vi "ME_acquire_10.vi"() -> ()   [LabVIEW 2015]
doc: "Use this template to build a producer/consumer design pattern. Use this template when you need to execute a process, such as data analysis, when a data source, such as a triggered acquisition, produces data at an uneven rate and you need to execute the process when the data becomes available."
uses:
  Mode.ctl
  oxford_driver/Oxford Drivers/BUSGEN.LLB/OxfordAddress.ctl
  <vilib>/Analysis/baseanly.llb/Mean (DBL).vi
  <vilib>/Utility/file.llb/Write Delimited Spreadsheet (DBL).vi
  <vilib>/express/express arith-compare/Formula/XNode/ExpressFormulaBlockNode.xnode
  <vilib>/Analysis/NI_AALBase.lvlib
panel:
  out "remaining elements":T1(array[cluster])
  in  "Stop":bool
  out "SaveSweep":bool=TRUE
  out "Measurement File_dn":path
  out "Measurement File_up":path
  out "Measurement File_average":path
  out "Actual Polarization":dbl
  in  "Reset IB?":bool
  in  "First?":bool
  in  "Save Period":dbl=1.0
  out "Averaged I(B)":dbl[][](array[numeric])
  out "P(uC/mm^2)":dbl[](array[numeric])
  in  "Sweep":bool
  out "P(B)":cluster{"yi":dbl[], dbl[]}(graph)
  out "Offset array":dbl[](array[numeric])
  in  "stop 2":bool
  in  "dB":dbl=0.005
  in  "Dwell Time (ms)":u32=1
  out "appended array":dbl[][](array[numeric])
  in  "Magnet ON?":bool
  out "Actual B Field (T)":dbl
  out "Actual Temperature (K)":dbl
  out "Actual Current (pA)":dbl
  in  "Tab Control":T2(tab)
  in  "Max temperature (K)":dbl=20.0
  in  "Min Temperature (K)":dbl=4.5
  out "P(T)":cluster{"yi":dbl[], dbl[]}(graph)
  out "I(T)":cluster{dbl[], dbl[]}(graph)
  in  "Set temperature (K)":dbl=4.5
  in  "Temp Ramping Rate (K/min)":dbl=10.0
  in  "Heater Range":enum16{"Off", "Low", "Medium", "High"}(ring)
  in  "Heater On/Off":bool
  out "Setpoint Temperature (K)":dbl
  in  "FileName":string
  out "Step Temp":bool
  out "j":i32
  out "i":i32
  in  "Max Countl":i32
  in  "Record ALL":bool
  in  "Sweep Rate Array":dbl[](array[numeric])=[2.0, 1.0, 0.5, 0.1, 0.05, 9.0, 10.0, 11.0, 12.0]
  out "I(B) 3":cluster{dbl[], dbl[]}[](graph)
  in  "Go to Set":bool
  in  "Set Field (T)":dbl
  in  "Field To Zero":bool
  in  "Sweep Rate (T/min)":dbl=2.0 format="%.6f"
  in  "Min Field (T)":dbl
  in  "Max Field (T)":dbl=0.15
  out "Up/Down":bool
  out "I(B) /Averaged/ 2":cluster{"B array":dbl[], dbl[]}[](graph)
  in  "Temperature Array":dbl[](array[numeric])=[4.5, 5.0, 6.0, 7.0, 8.0, 9.0, 10.0, 11.0, 12.0]
  out "New":bool=TRUE
  out "Step Rate":bool
  out "Finished":bool=TRUE
  in  "Directory":string
  out "Wait (s)":dbl
  in  "secs to wait":dbl=180.0
  in  "Max count array":i32[](array[numeric])=[2, 1, 0, 0, 0, 9, 10, 11, 12]
  in  "Measure Noise":bool
  in  "Cycles":i32
  in  "maximum value":dbl=10.0 format="%0.2f"
  in  "minimum value":dbl=-10.0 format="%0.2f"
  in  "physical channels":tag="Dev1/ai1"
  out "PSD (pA/Hz^1/2) Peaks Removed":cluster{"f0":dbl, "df":dbl, "magnitude":dbl[]}(graph)
  out "PSD (pA/Hz^1/2)":cluster{"f0":dbl, "df":dbl, "magnitude":dbl[]}(graph)
  out "Current (pA) Filtered":waveform(dbl)(graph)
  out "Current (pA)":dbl[](graph)
  in  "Samples per channel":i32=1000
  in  "Rate":dbl=1000.0 format="%0.2f"
  in  "Cut-Off Frequency":dbl=100.0 caption="Lower Cut-Off"
  in  "Filter On":bool
  out "Dc offset":dbl
  in  "Calibrate":bool
  in  "IV converter":refnum<visa-resource-name>="GPIB0::20::INSTR"
  in  "Magnetic Field":refnum<visa-resource-name>="GPIB0::21::INSTR"
  out "Time Lag":dbl=0.0500025749206543
  in  "Lake Shore":refnum<visa-resource-name>="GPIB0::11::INSTR"
  in  "Temp Refresh (s)":dbl=0.1
  in  "Sampling rate (Hz)":dbl=10.0
  in  "Gain (V/A)":dbl=1000000000.0
  in  "Sample area (mm^2)":dbl=3.9
  out "B_V":cluster{dbl[], "Best Linear Fit":dbl[]}[](graph)=[{[-0.00854253601, 0.00626134724, 0.0219834428, 0.0379117736, 0.0535871506, 0.0694316728, 0.0851615152, 0.100816481, 0.116478038, 0.132148461, 0.147876163, 0.16341701, 0.178976744, 0.194563632, 0.210251739, 0.225738944, 0.241298253, 0.256806034, 0.272344374, 0.287933477, 0.303494709, 0.318997125, 0.334591297, 0.350146681, 0.365618053, 0.380940961, 0.39666457, 0.412213675, 0.427724671, 0.443221444, 0.458760641, 0.474360042, 0.489915118, 0.505330598, 0.520967119, 0.536347531, 0.551813711, 0.567441155, 0.582995861, 0.598507522, 0.614041988, 0.629563151, 0.645106262, 0.660611914, 0.676136149, 0.691553948, 0.7071244, 0.72262999, 0.738171137, 0.753700392, 0.76919513, 0.784778028, 0.800215944, 0.8156961, 0.831325434, 0.846852183, 0.862326812, 0.877819169, 0.893312568, 0.90888536, 0.924354789], "Best Linear Fit"=[0.0, 0.005, 0.01, 0.015, 0.02, 0.025, 0.03, 0.035, 0.04, 0.045, 0.05, 0.055, 0.06, 0.065, 0.07, 0.075, 0.08, 0.085, 0.09, 0.095, 0.1, 0.105, 0.11, 0.115, 0.12, 0.125, 0.13, 0.135, 0.14, 0.145, 0.15, 0.155, 0.16, 0.165, 0.17, 0.175, 0.18, 0.185, 0.19, 0.195, 0.2, 0.205, 0.21, 0.215, 0.22, 0.225, 0.23, 0.235, 0.24, 0.245, 0.25, 0.255, 0.26, 0.265, 0.27, 0.275, 0.28, 0.285, 0.29, 0.295, 0.3]}, {[-0.00854253601, 0.00626134724, 0.0219834428, 0.0379117736, 0.0535871506, 0.0694316728, 0.0851615152, 0.100816481, 0.116478038, 0.132148461, 0.147876163, 0.16341701, 0.178976744, 0.194563632, 0.210251739, 0.225738944, 0.241298253, 0.256806034, 0.272344374, 0.287933477, 0.303494709, 0.318997125, 0.334591297, 0.350146681, 0.365618053, 0.380940961, 0.39666457, 0.412213675, 0.427724671, 0.443221444, 0.458760641, 0.474360042, 0.489915118, 0.505330598, 0.520967119, 0.536347531, 0.551813711, 0.567441155, 0.582995861, 0.598507522, 0.614041988, 0.629563151, 0.645106262, 0.660611914, 0.676136149, 0.691553948, 0.7071244, 0.72262999, 0.738171137, 0.753700392, 0.76919513, 0.784778028, 0.800215944, 0.8156961, 0.831325434, 0.846852183, 0.862326812, 0.877819169, 0.893312568, 0.90888536, 0.924354789], "Best Linear Fit"=[-0.00022554388023060128, 0.004536267537808887, 0.009593430775915074, 0.014716931562355689, 0.01975906732634002, 0.024855610270593523, 0.029915265354287977, 0.03495083565949541, 0.03998852608757118, 0.045029068349812316, 0.05008803495326229, 0.055086897848955874, 0.060091835929837946, 0.06510550835596321, 0.07015173884687344, 0.07513334727738563, 0.08013814865293042, 0.08512637555172443, 0.0901244320467579, 0.09513881694893507, 0.10014423687592358, 0.10513073807087174, 0.11014675346564809, 0.1151502923271957, 0.12012680792099008, 0.1250555686413888, 0.1301132186920259, 0.13511473785283767, 0.14010399888730068, 0.14508868495702945, 0.1500870171143548, 0.15510471446726903, 0.16010815425765457, 0.16506669165212906, 0.17009632901003072, 0.1750435864450521, 0.18001843198211442, 0.1850451496356715, 0.19004847041199868, 0.1950379453501071, 0.20003475573578386, 0.20502728708357412, 0.21002687821664084, 0.21501442030211, 0.220007939788244, 0.2249672231113706, 0.22997560874002893, 0.23496313088260184, 0.23996209027618054, 0.24495722449359253, 0.24994125598600042, 0.2549536449902534, 0.25991939913989753, 0.2648987401917687, 0.26992606578200207, 0.2749203939204135, 0.2798979571595809, 0.2848812227804405, 0.2898648235706211, 0.2948739618827834, 0.2998498524919418]}]
  out "V_I":cluster{dbl[], "Best Linear Fit":dbl[]}[](graph)=[{[0.0, 0.035, 0.069, 0.104, 0.138, 0.173, 0.208, 0.242, 0.277, 0.311, 0.346, 0.38, 0.415, 0.45, 0.484, 0.519, 0.553, 0.588, 0.623, 0.657, 0.692, 0.726, 0.761, 0.796, 0.83, 0.865, 0.899, 0.934, 0.969, 1.003, 1.038, 1.072, 1.107, 1.141, 1.176, 1.211, 1.245, 1.28, 1.314, 1.349, 1.384, 1.418, 1.453, 1.487, 1.522, 1.557, 1.591, 1.626, 1.66, 1.695, 1.73, 1.764, 1.799, 1.833, 1.868, 1.902, 1.937, 1.972, 2.006, 2.041, 2.075], "Best Linear Fit"=[-0.00854253601, 0.00626134724, 0.0219834428, 0.0379117736, 0.0535871506, 0.0694316728, 0.0851615152, 0.100816481, 0.116478038, 0.132148461, 0.147876163, 0.16341701, 0.178976744, 0.194563632, 0.210251739, 0.225738944, 0.241298253, 0.256806034, 0.272344374, 0.287933477, 0.303494709, 0.318997125, 0.334591297, 0.350146681, 0.365618053, 0.380940961, 0.39666457, 0.412213675, 0.427724671, 0.443221444, 0.458760641, 0.474360042, 0.489915118, 0.505330598, 0.520967119, 0.536347531, 0.551813711, 0.567441155, 0.582995861, 0.598507522, 0.614041988, 0.629563151, 0.645106262, 0.660611914, 0.676136149, 0.691553948, 0.7071244, 0.72262999, 0.738171137, 0.753700392, 0.76919513, 0.784778028, 0.800215944, 0.8156961, 0.831325434, 0.846852183, 0.862326812, 0.877819169, 0.893312568, 0.90888536, 0.924354789]}, {[0.0, 0.035, 0.069, 0.104, 0.138, 0.173, 0.208, 0.242, 0.277, 0.311, 0.346, 0.38, 0.415, 0.45, 0.484, 0.519, 0.553, 0.588, 0.623, 0.657, 0.692, 0.726, 0.761, 0.796, 0.83, 0.865, 0.899, 0.934, 0.969, 1.003, 1.038, 1.072, 1.107, 1.141, 1.176, 1.211, 1.245, 1.28, 1.314, 1.349, 1.384, 1.418, 1.453, 1.487, 1.522, 1.557, 1.591, 1.626, 1.66, 1.695, 1.73, 1.764, 1.799, 1.833, 1.868, 1.902, 1.937, 1.972, 2.006, 2.041, 2.075], "Best Linear Fit"=[-0.007846580254753975, 0.007882153481927697, 0.02316149482613275, 0.03889022856281441, 0.054169569907019474, 0.06989830364370113, 0.08562703738038281, 0.10090637872458785, 0.11663511246126955, 0.1319144538054746, 0.14764318754215625, 0.1629225288863613, 0.17865126262304296, 0.19437999635972467, 0.2096593377039297, 0.22538807144061138, 0.24066741278481643, 0.25639614652149806, 0.27212488025817977, 0.2874042216023848, 0.3031329553390665, 0.31841229668327153, 0.3341410304199532, 0.3498697641566349, 0.3651491055008399, 0.3808778392375216, 0.39615718058172666, 0.4118859143184083, 0.42761464805509, 0.442893989399295, 0.45862272313597674, 0.4739020644801818, 0.48963079821686345, 0.5049101395610684, 0.5206388732977502, 0.5363676070344319, 0.5516469483786369, 0.5673756821153185, 0.5826550234595236, 0.5983837571962053, 0.6141124909328869, 0.629391832277092, 0.6451205660137737, 0.6603999073579787, 0.6761286410946604, 0.691857374831342, 0.7071367161755471, 0.7228654499122288, 0.7381447912564338, 0.7538735249931156, 0.7696022587297972, 0.7848816000740022, 0.8006103338106839, 0.815889675154889, 0.8316184088915707, 0.8468977502357756, 0.8626264839724573, 0.878355217709139, 0.893634559053344, 0.9093632927900257, 0.9246426341342309]}]
  out "B0 (T)":dbl=0.0025222449819540214
  out "B/V (T/V)":dbl=0.321659617116981
  out "I0 (A)":dbl=-0.007846580254753975
  out "V/I (Ohm)":dbl=0.44939239247661916
  in  "Offset?":bool
  in  "Temp/Magnetic Field":bool
  out "index":i8
  out "Read?":bool
  out "Magnetic Field (T)":dbl[](array[numeric])
  out "Reset":bool
  out "Measured Current (pA)":dbl[](array[numeric])
  out "Elapsed Time (s)":dbl[](array[numeric])
  out "Start time":timestamp
  in  "Enum":T3=enum."Process"
  out "B array":dbl[](array[numeric])
  in  "dB (T)":dbl=0.0025
  in  "Counter":i8
  out "L magnet (H)":dbl
  out "R magnet (mOhm)":dbl
  out "Actual Current (R0)":dbl
  out "Actual Field (T)":dbl
  out "Temperature array":dbl[](array[numeric])
  in  "New Measurement File":bool
  out "Measurement File":path
  out "refnum out":refnum<file>
  in  "Measuring":bool
  in  "Measure /Pause":bool
  in  "stop":bool
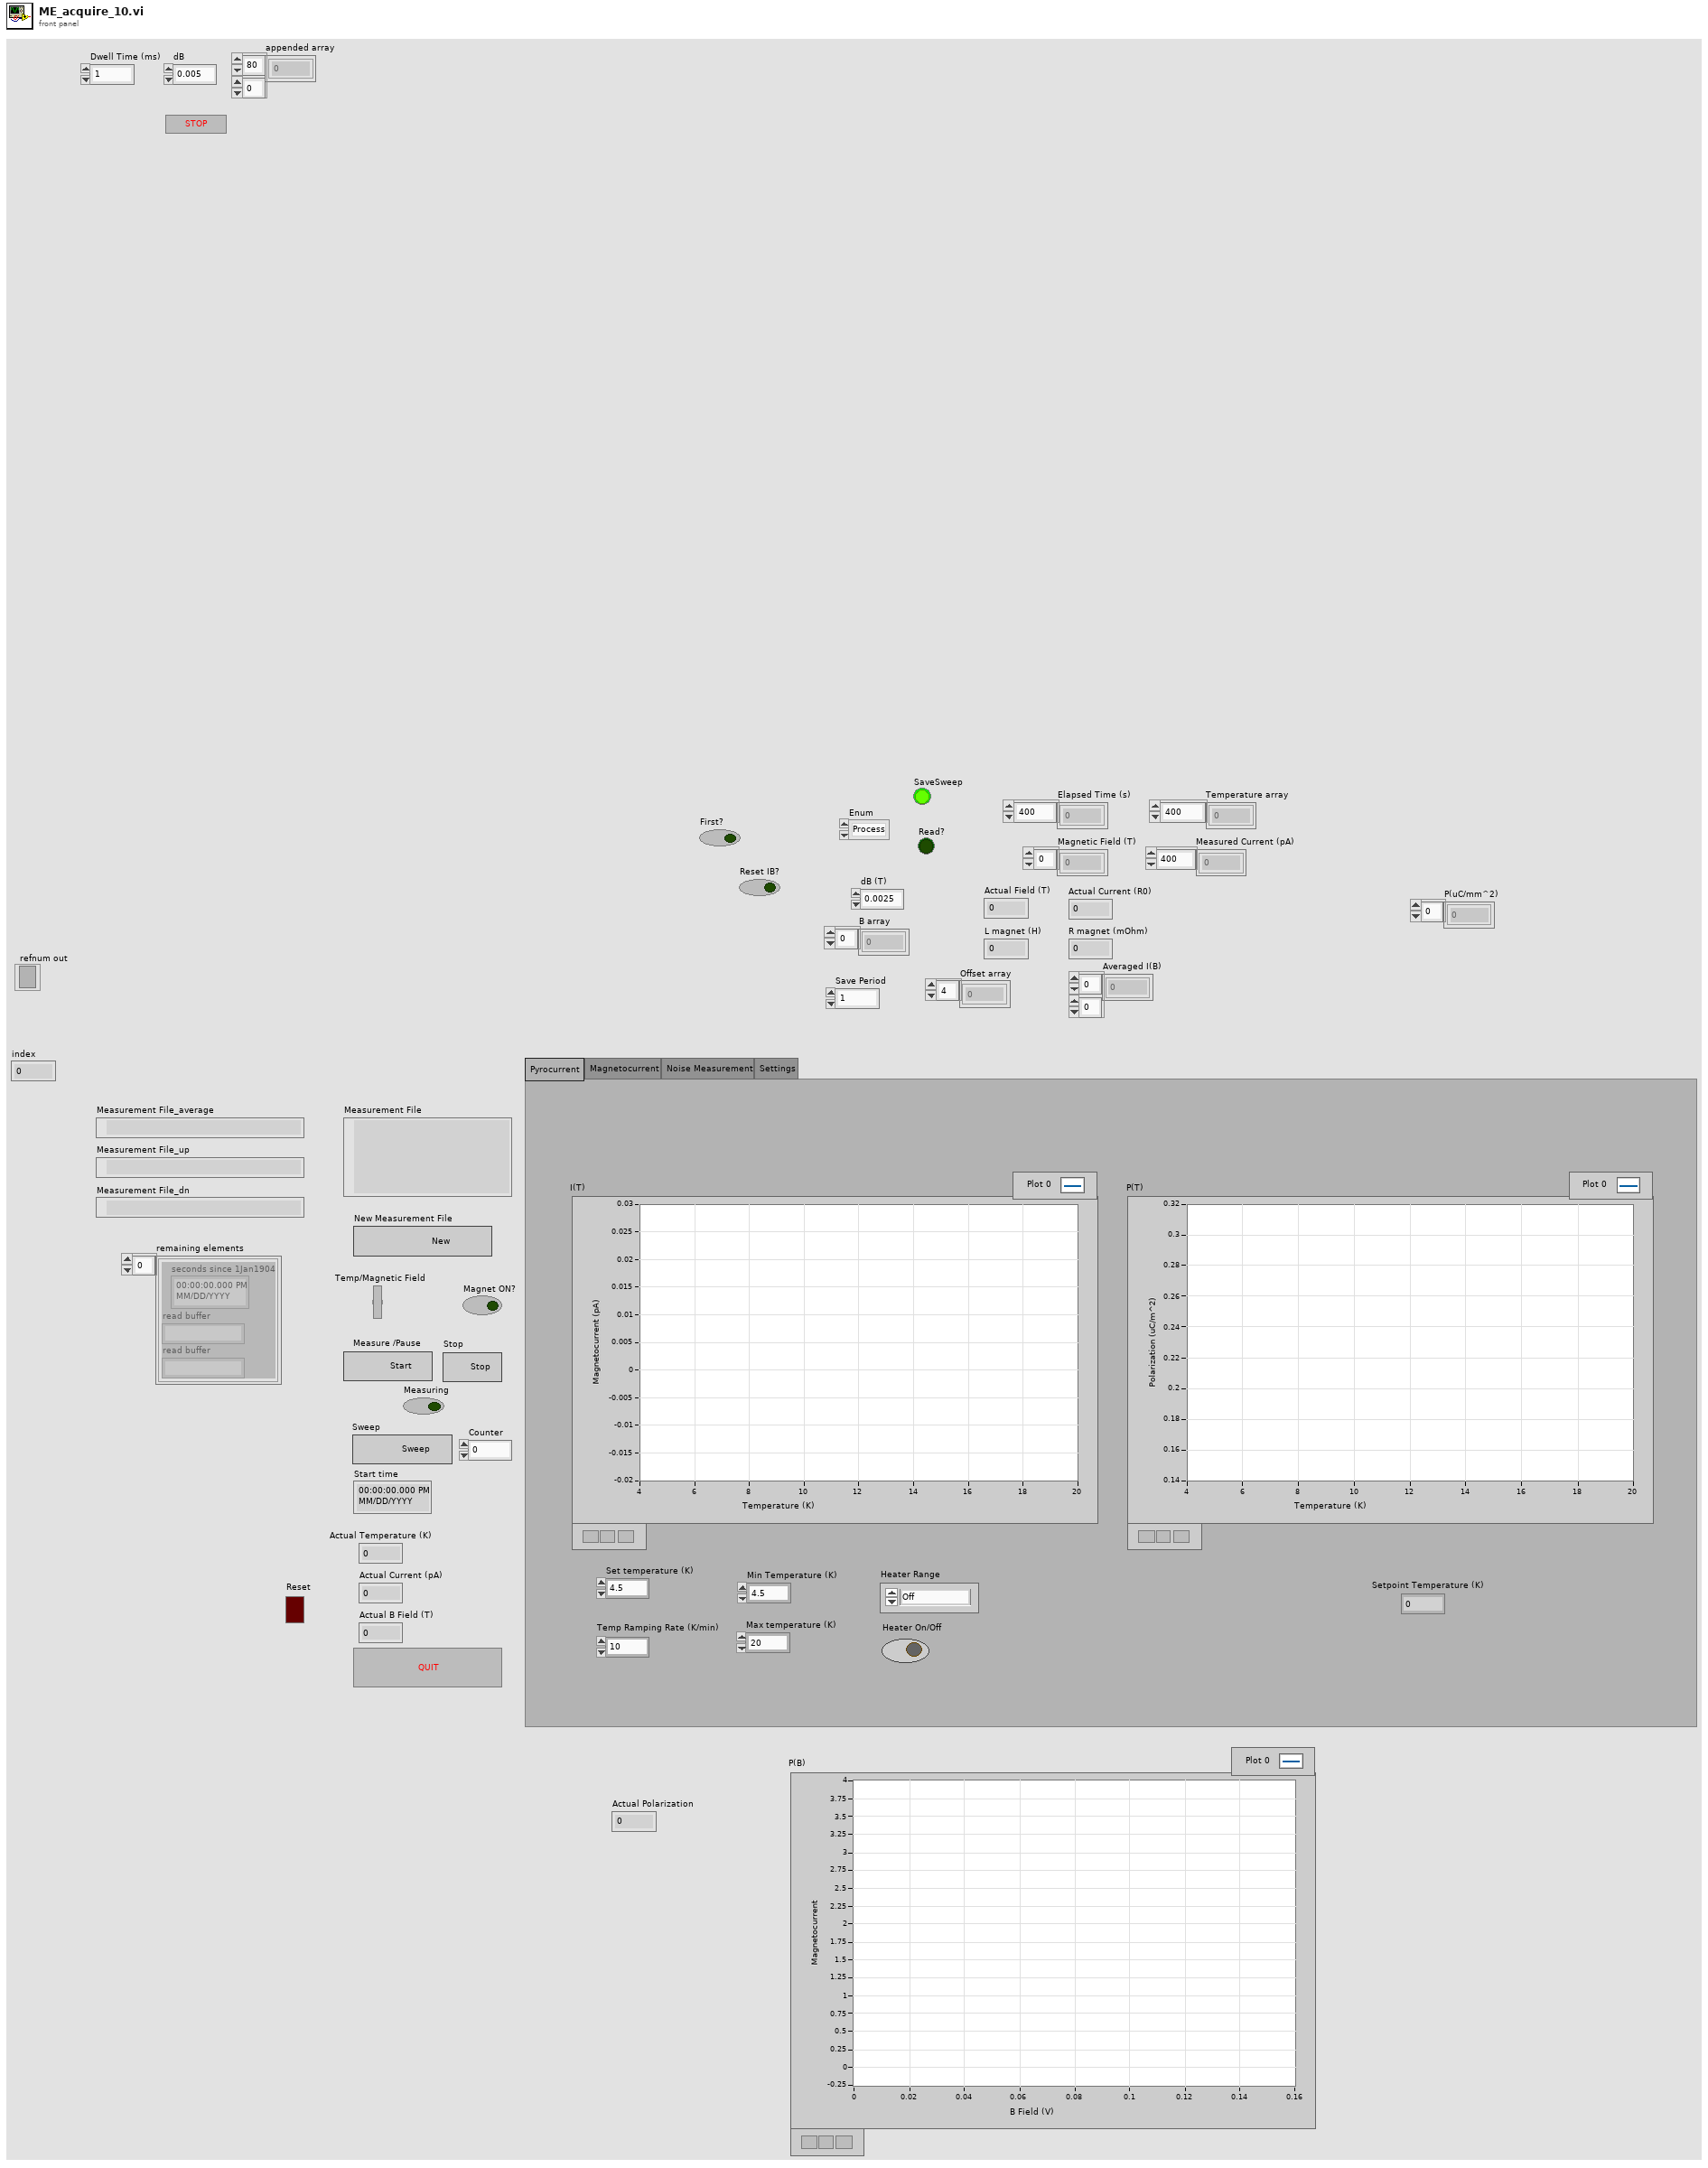
[diagram p1: front panel]
types:
  T1 = cluster{"seconds since 1Jan1904":timestamp, "read buffer":string, "read buffer":string}[]
  T2 = enum32{"Pyrocurrent", "Magnetocurrent", "Noise Measurement", "Settings"}
  T3 = typedef "Mode.ctl" = enum16{"Offset", "Process", "Sweep", "Plot", "Save", "New", "Return", ""}
  T4 = enum16{"open", "replace", "create", "open or create", "replace or create", "replace or create with confirmation"}
  T5 = typedef "OxfordAddress.ctl" = cluster{"Com Port":i32, "ISOBUS Address":i32, "GPIB Address":i16, "Communication":enum16{"RS232", "ISOBUS", "GPIB", "Gateway"}}
  T6 = cluster{"seconds since 1Jan1904":timestamp, "read buffer":string, "read buffer":string}
  T7 = cluster{"B array":dbl[], "Averaged I(B) out":dbl[]}
  T8 = cluster{"B array":dbl[], "Averaged I(B) out":dbl[]}[]
  T9 = cluster{"I array out (A)":dbl[], "V array out (V)":dbl[]}
  T10 = cluster{"I array out (A)":dbl[], "Best Linear Fit":dbl[]}
  T11 = cluster{"V array out (V)":dbl[], "B array Out":dbl[]}
  T12 = cluster{"V array out (V)":dbl[], "Best Linear Fit 2":dbl[]}
  T13 = cluster{"I array out (A)":dbl[], "Best Linear Fit":dbl[]}[]
  T14 = cluster{"V array out (V)":dbl[], "Best Linear Fit 2":dbl[]}[]
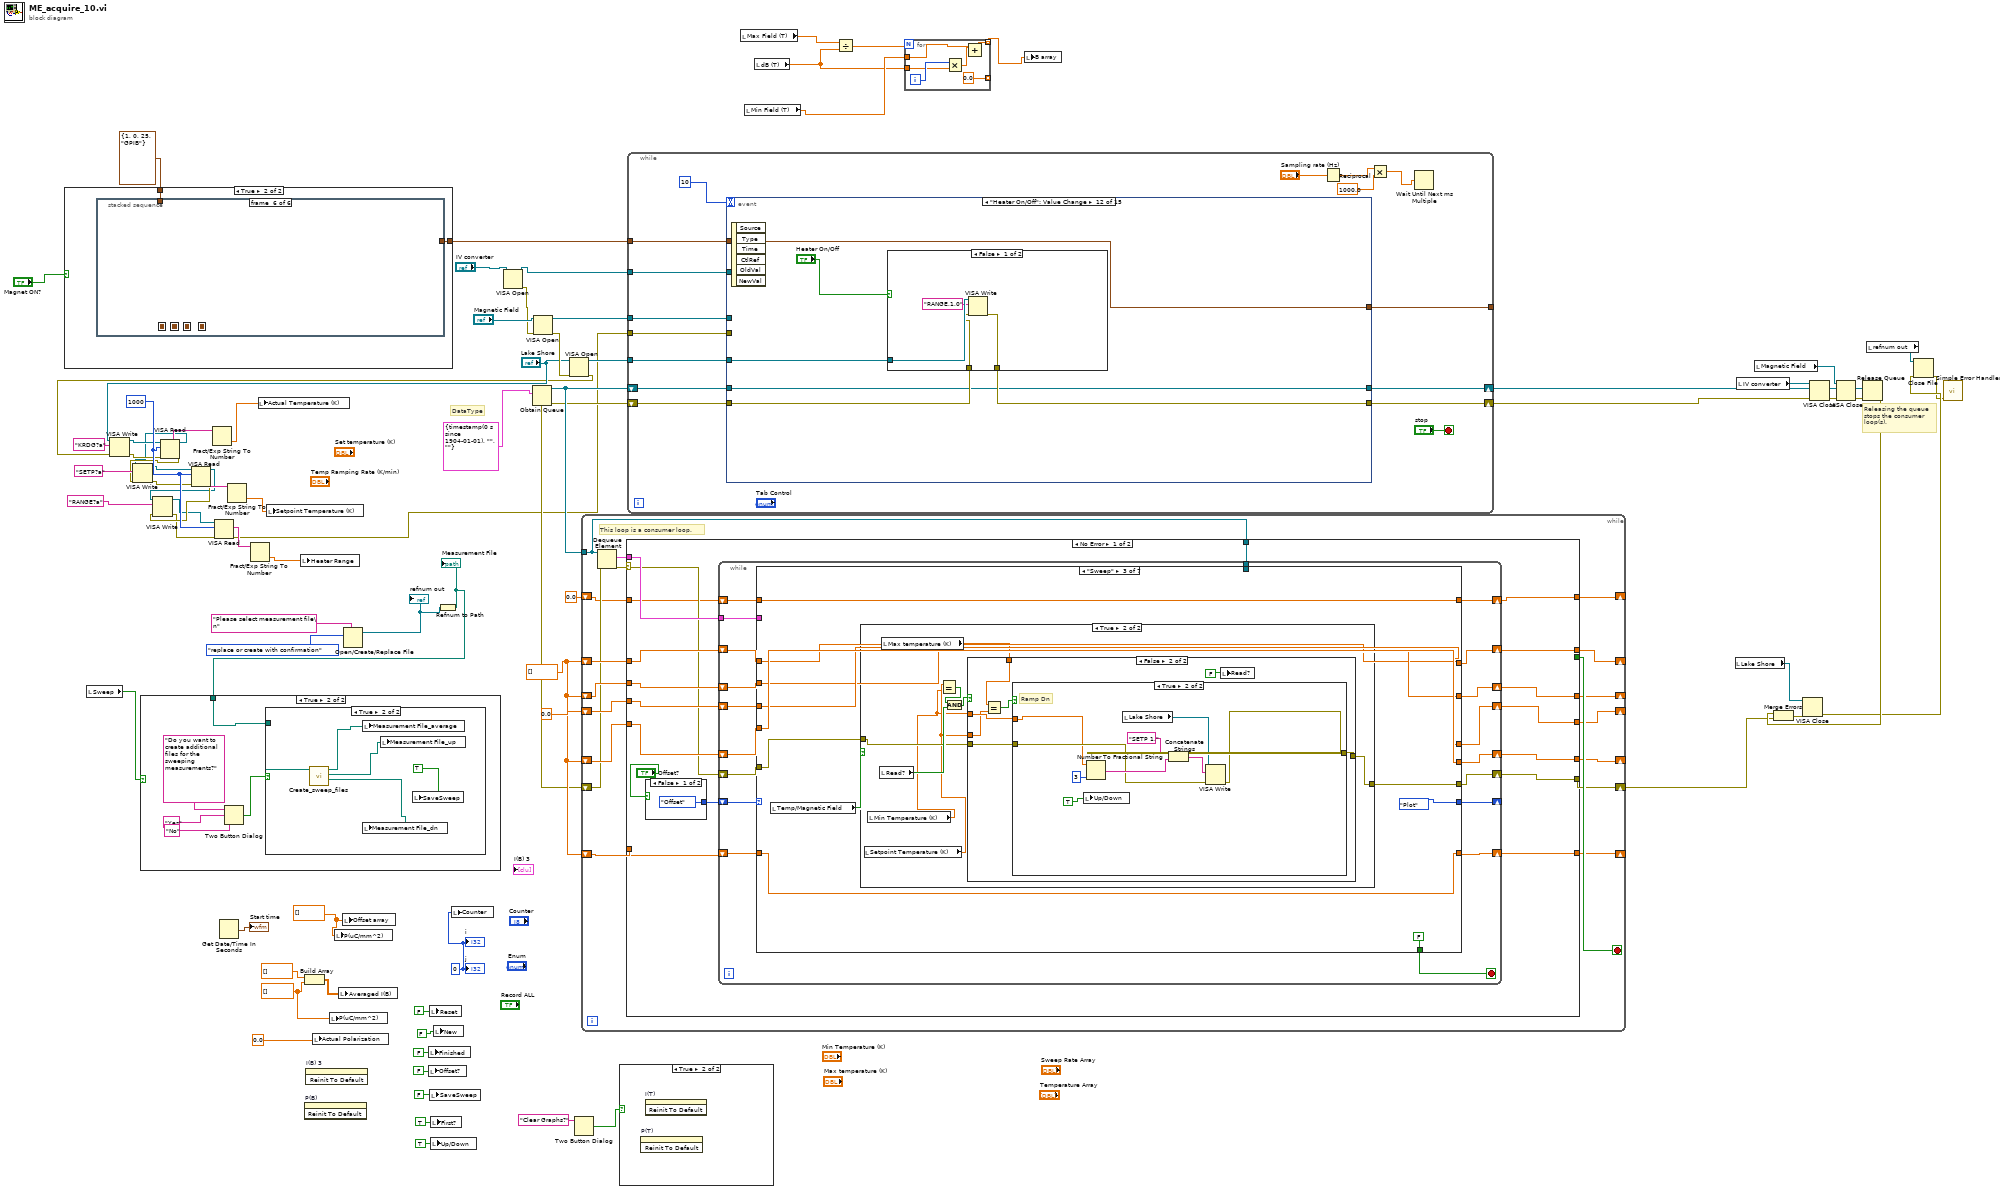
[diagram p0: block diagram]
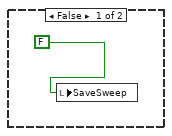
[diagram p4: hidden frame]
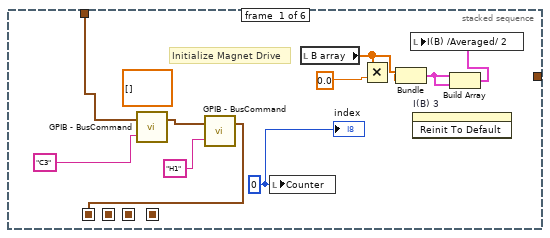
[diagram p6: hidden frame]
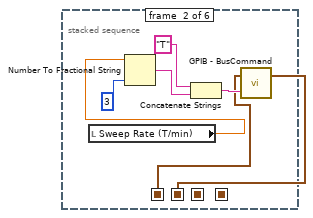
[diagram p7: hidden frame]
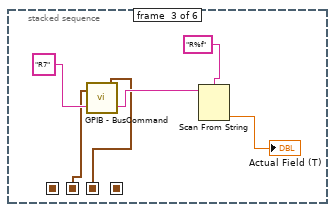
[diagram p8: hidden frame]
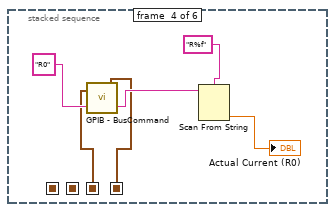
[diagram p9: hidden frame]
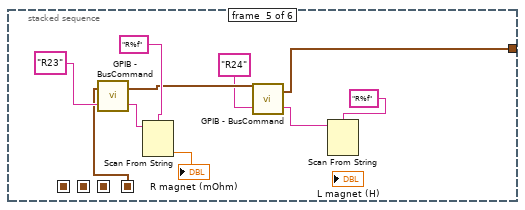
[diagram p10: hidden frame]
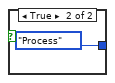
[diagram p11: hidden frame]
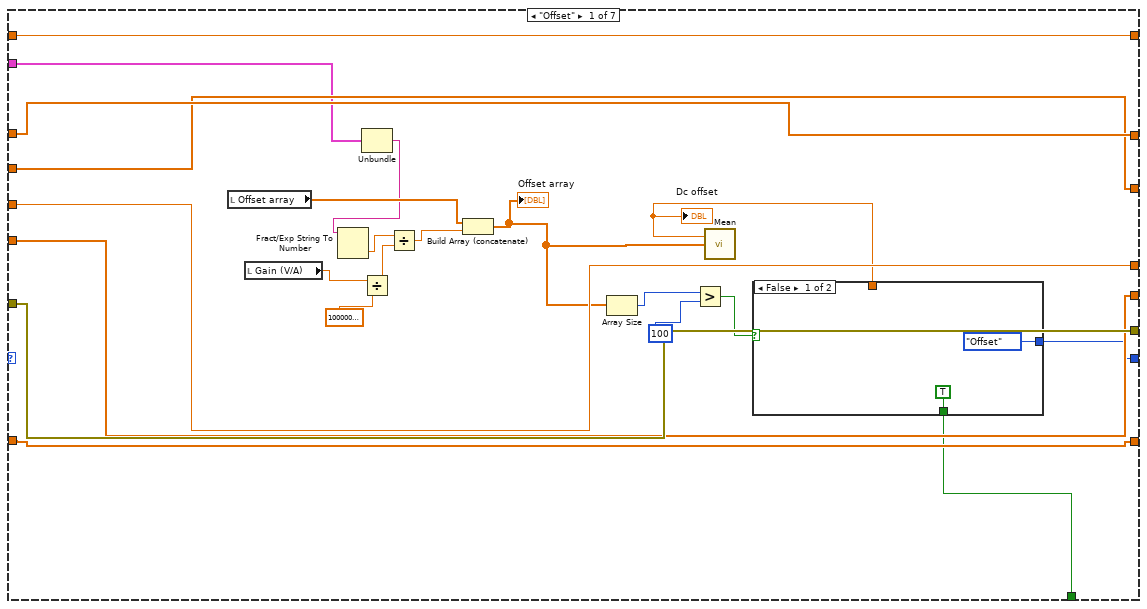
[diagram p12: hidden frame]
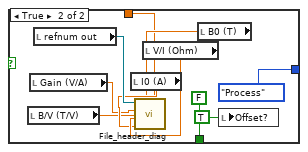
[diagram p13: hidden frame]
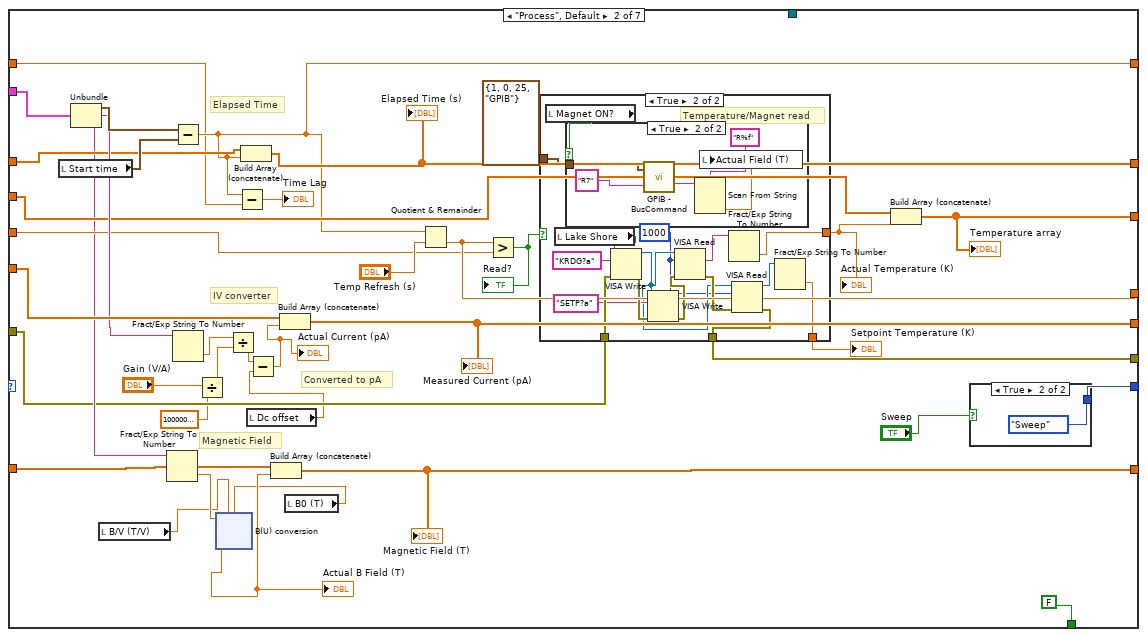
[diagram p14: hidden frame]
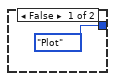
[diagram p15: hidden frame]
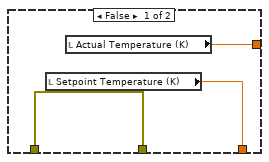
[diagram p16: hidden frame]
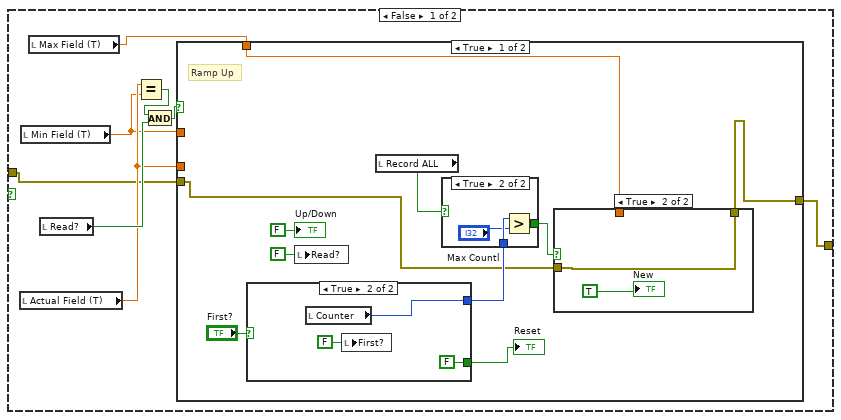
[diagram p18: hidden frame]
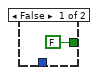
[diagram p19: hidden frame]
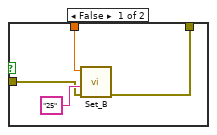
[diagram p20: hidden frame]
diagram:
  w16 = u32 1000 ("byte count")
  w27 = 0 ("j")
  w24 = dbl[] []
  w45 = dbl[] []
  w51 = dbl[] []
  # "DataType"
  # "Releasing the queue stops the consumer loop(s)."
  n1 = case shown="True" "Magnet ON?" {
    tunnel: T5 {"Com Port"=1, "ISOBUS Address"=0, "GPIB Address"=25, "Communication"=enum."GPIB"} ("Address") -> [w79 w81]
    tunnel: [w79 w80] -> w58
    frame False {
    }
    frame True {
      n2 = stacked-sequence {
        seq-local: [w89 _ _ _ _ _] -> [_ w94 _ _ _ _]
        seq-local: [_ w93 _ _ _ _] -> [_ _ w101 _ _ _]
        seq-local: [_ _ w100 _ _ _] -> [_ _ _ w107 _ _]
        seq-local: [_ _ _ w106 _ _] -> [_ _ _ _ w117 _]
        tunnel: w81 -> [w91 _ _ _ _ _]
        tunnel: [_ _ _ _ w115 _] -> w80
        frame #0 {
          (unwired) dbl[][] []
          w87 = i8 0 ("Counter")
          # "Initialize Magnet Drive"
          n3 = call "GPIB - BusCommand.vi"("Command"="C3", "Address"=w91) -> ("Address(thru)"=w90:T5)  [unwired: 1 out]
          n4 = call "GPIB - BusCommand.vi"("Command"="H1", "Address"=w90) -> ("Address(thru)"=w89:T5)  [unwired: 1 out]
          n5 = local write "Counter"(w87) -> ()
          n6 = local read "B array"() -> (w85:dbl[])
          n7 = Multiply(x=w85, y=0.0) -> (x*y=w84:dbl[])
          n8 = Bundle("B array"=w85, w84) -> (w83:cluster{"B array":dbl[], dbl[]})  [unwired: 1 in]
          n9 = invoke on="I(B) 3" class="XYGraph (strict)" method="Reinit To Default"() -> ()  [unwired: 3 in, 3 out]
          n10 = Build Array(w83, w83) -> (w82:cluster{"B array":dbl[], dbl[]}[])
          n11 = local write "I(B) /Averaged/ 2"(w82) -> ()
          "index" <- w87
        }
        frame #1 {
          n12 = local read "Sweep Rate (T/min)"() -> (w95:dbl)
          n13 = Number To Fractional String(number=w95, precision (6)=i16 3) -> (F-format string=w97:string)  [unwired: 2 in]
          n14 = Concatenate Strings("T" ("format string"), w97) -> (w96:string)
          n15 = call "GPIB - BusCommand.vi"("Command"=w96, "Address"=w94) -> ("Address(thru)"=w93:T5)  [unwired: 1 out]
        }
        frame #2 {
          n16 = call "GPIB - BusCommand.vi"("Command"="R7" ("format string"), "Address"=w101) -> ("Reply"=w105:string, "Address(thru)"=w100:T5)
          n17 = Scan From String(format string="R%f" ("remaining string"), input string=w105) -> (output 1=→"Actual Field (T)":dbl)  [unwired: 3 in, 3 out]
        }
        frame #3 {
          n18 = call "GPIB - BusCommand.vi"("Command"="R0" ("format string"), "Address"=w107) -> ("Reply"=w111:string, "Address(thru)"=w106:T5)
          n19 = Scan From String(format string="R%f" ("remaining string"), input string=w111) -> (output 1=→"Actual Current (R0)":dbl)  [unwired: 3 in, 3 out]
        }
        frame #4 {
          n20 = call "GPIB - BusCommand.vi"("Command"="R23" ("format string"), "Address"=w117) -> ("Reply"=w121:string, "Address(thru)"=w116:T5)
          n21 = Scan From String(format string="R%f" ("remaining string"), input string=w121) -> (output 1=→"R magnet (mOhm)":dbl)  [unwired: 3 in, 3 out]
          n22 = call "GPIB - BusCommand.vi"("Command"="R24" ("format string"), "Address"=w116) -> ("Reply"=w113:string, "Address(thru)"=w115:T5)
          n23 = Scan From String(format string="R%f" ("remaining string"), input string=w113) -> ()  [unwired: 4 in, 3 out]
        }
        frame #5 {
        }
      }
    }
  }
  n24 = local read "Sweep"() -> (w32:bool)
  n25 = Get Date/Time In Seconds() -> (seconds since 1Jan1904=→"Start time":timestamp)
  n26 = Build Array(dbl[] [], w24) -> (w43:dbl[][])
  n27 = invoke on="P(B)" class="XYGraph (strict)" method="Reinit To Default"() -> ()  [unwired: 3 in, 3 out]
  n28 = invoke on="I(B) 3" class="XYGraph (strict)" method="Reinit To Default"() -> ()  [unwired: 3 in, 3 out]
  n29 = local write "Actual Polarization"(0.0 ("Actual Polarization")) -> ()
  n30 = local write "P(uC/mm^2)"(w24) -> ()
  n31 = local write "P(uC/mm^2)"(w45) -> ()
  n32 = local write "Averaged I(B)"(w43) -> ()
  n33 = local write "Offset array"(w45) -> ()
  n34 = Open/Create/Replace File(prompt="Please select measurement file\n", operation (0:open)=T4."replace or create with confirmation") -> (refnum out=w55:refnum<file>)  [unwired: 4 in, 2 out]
  "refnum out" <- w55
  n35 = local write "Finished"(FALSE ("Finished")) -> ()
  n36 = local write "Offset?"(FALSE ("Offset?")) -> ()
  n37 = local write "Reset"(FALSE ("Reset")) -> ()
  n38 = local write "SaveSweep"(FALSE ("SaveSweep")) -> ()
  n39 = local write "First?"(TRUE ("First?")) -> ()
  n40 = local write "Up/Down"(TRUE ("Up/Down")) -> ()
  n41 = local write "New"(FALSE ("New")) -> ()
  n42 = Refnum to Path(1:w55) -> (0:w31:path)
  "Measurement File" <- w31
  n43 = case shown="True" w32 {
    tunnel: w31 -> [_ w122]
    frame False {
    }
    frame True {
      n44 = Two Button Dialog(message="Do you want to create additional files for the sweeping measurements?" ("string"), 1:"No" ("F button name (\"Cancel\")"), 2:"Yes" ("T button name (\"OK\")")) -> (T button?=w124:bool)
      n45 = case shown="True" w124 {
        tunnel: w122 -> [_ w132]
        frame False {
          n46 = local write "SaveSweep"(FALSE ("SaveSweep")) -> ()
        }
        frame True {
          n47 = call "Create_sweep_files.vi"("Measurement File"=w132) -> ("Path 3"=w129:path, "Path 2"=w130:path, "Path"=w131:path)  [unwired: 8 in]
          n48 = local write "Measurement File_dn"(w129) -> ()
          n49 = local write "Measurement File_average"(w131) -> ()
          n50 = local write "Measurement File_up"(w130) -> ()
          n51 = local write "SaveSweep"(TRUE) -> ()
        }
      }
    }
  }
  n52 = local write "Counter"(w27) -> ()
  n53 = VISA Open(VISA resource name="IV converter") -> (VISA resource name=w73:refnum<visa-resource-name>, error out=w75:errorcluster)  [unwired: 4 in]
  n54 = Obtain Queue(element data type=T6 {"seconds since 1Jan1904"=timestamp(0 s since 1904-01-01), "read buffer"="", "read buffer"=""} ("output cluster")) -> (queue out=w78:refnum<queue>, error out=w49:errorcluster)  [unwired: 4 in, 1 out]
  n55 = VISA Open(error in (no error)=w75, VISA resource name="Magnetic Field") -> (VISA resource name=w72:refnum<visa-resource-name>, error out=w52:errorcluster)  [unwired: 3 in]
  n56 = VISA Open(error in (no error)=w52, VISA resource name="Lake Shore") -> (VISA resource name=w47:refnum<visa-resource-name>, error out=w13:errorcluster)  [unwired: 3 in]
  n57 = VISA Write(VISA resource name="Lake Shore", write buffer="KRDG?a", error in (no error)=w13) -> (VISA resource name out=w10:refnum<visa-resource-name>, error out=w9:errorcluster)  [unwired: 1 out]
  n58 = VISA Read(VISA resource name=w10, byte count=w16, error in (no error)=w9) -> (VISA resource name out=w7:refnum<visa-resource-name>, read buffer=w21:string, error out=w8:errorcluster)  [unwired: 1 out]
  n59 = VISA Write(VISA resource name=w7, write buffer="SETP?a", error in (no error)=w8) -> (VISA resource name out=w6:refnum<visa-resource-name>, error out=w5:errorcluster)  [unwired: 1 out]
  n60 = VISA Read(VISA resource name=w6, byte count=w16, error in (no error)=w5) -> (VISA resource name out=w3:refnum<visa-resource-name>, read buffer=w20:string, error out=w4:errorcluster)  [unwired: 1 out]
  n61 = VISA Write(VISA resource name=w3, write buffer="RANGE?a", error in (no error)=w4) -> (VISA resource name out=w1:refnum<visa-resource-name>, error out=w2:errorcluster)  [unwired: 1 out]
  n62 = Fract/Exp String To Number(string=w21) -> (number=w19:dbl)  [unwired: 3 in, 1 out]
  n63 = VISA Read(VISA resource name=w1, byte count=w16, error in (no error)=w2) -> (read buffer=w15:string, error out=w12:errorcluster)  [unwired: 2 out]
  n64 = Fract/Exp String To Number(string=w20) -> (number=w18:dbl)  [unwired: 3 in, 1 out]
  n65 = Fract/Exp String To Number(string=w15) -> (number=w11:dbl)  [unwired: 3 in, 1 out]
  n66 = local write "Actual Temperature (K)"(w19) -> ()
  n67 = local write "Setpoint Temperature (K)"(w18) -> ()
  n68 = local write "Heater Range"(w11) -> ()
  n69 = Two Button Dialog(message="Clear Graphs?") -> (T button?=w26:bool)  [unwired: 2 in]
  n70 = while {
    tunnel: w78 -> [w133]
    shift-right: [w146] -> _
    shift-left: w51 -> [w145]
    shift-right: [w144] -> _
    shift-left: w51 -> [w143]
    shift-right: [w142] -> _
    shift-left: w51 -> [w141]
    shift-right: [w140] -> _
    shift-left: 0.0 -> [w139]
    shift-right: [w138] -> _
    shift-left: w51 -> [w137]
    shift-right: [w147] -> w63
    shift-left: w49 -> [w136]
    shift-right: [w135] -> _
    shift-left: 0.0 -> [w134]
    stop <- w148 stop-if-true
    # "This loop is a consumer loop."
    n71 = Dequeue Element(queue=w133, error in (no error)=w136) -> (element=w149:T6, error out=w150:errorcluster)  [unwired: 1 in, 2 out]
    n72 = case shown="No Error" w150 {
      selector: w150 -> [w156 w714]
      tunnel: w149 -> [w167 _]
      tunnel: [_ TRUE] -> w148
      tunnel: [w155 w714] -> w147
      tunnel: [w166 w713] -> w146
      tunnel: w145 -> [w165 w713]
      tunnel: [w164 w710] -> w144
      tunnel: w143 -> [w163 w710]
      tunnel: [w162 w709] -> w142
      tunnel: w141 -> [w161 w709]
      tunnel: [w160 w711] -> w140
      tunnel: w139 -> [w159 w711]
      tunnel: [w158 w712] -> w138
      tunnel: w137 -> [w157 w712]
      tunnel: [w154 w708] -> w135
      tunnel: w134 -> [w153 w708]
      tunnel: w133 -> [w151 _]
      frame No Error {
        n73 = case shown="False" "Offset?" {
          tunnel: [Mode."Offset" ("Enum") Mode."Process" ("Enum")] -> w168
          frame False {
          }
          frame True {
          }
        }
        n74 = while {
          shift-right: [w177] -> _
          shift-left: w168 -> [w189]
          tunnel: w167 -> [w188]
          shift-right: [w187] -> w166
          shift-left: w165 -> [w186]
          shift-right: [w179] -> w158
          shift-left: w157 -> [w178]
          shift-right: [w181] -> w160
          shift-left: w159 -> [w180]
          shift-right: [w185] -> w164
          shift-left: w163 -> [w184]
          shift-right: [w175] -> w155
          shift-left: w156 -> [w176]
          shift-right: [w183] -> w162
          shift-left: w161 -> [w182]
          shift-right: [w173] -> w154
          shift-left: w153 -> [w172]
          tunnel: w151 -> [w171]
          stop <- w174 stop-if-true
          n75 = case shown="\"Sweep\"" w189 {
            selector: w189 -> [_ _ _ _ _ _ w701]
            tunnel: w188 -> [w205 w260 _ _ _ _ _]
            tunnel: [w211 w257 w304 w409 w482 w550 w706] -> w187
            tunnel: w186 -> [w211 w248 w304 w409 w478 w550 w706]
            tunnel: [w206 w256 w307 w411 w484 w548 w703] -> w185
            tunnel: w184 -> [w206 w255 w307 w411 w479 w548 w703]
            tunnel: [w207 w252 w309 w406 w485 w546 w700] -> w183
            tunnel: w182 -> [w207 w251 w309 w406 w480 w546 w700]
            tunnel: [w209 w247 w306 w407 w488 0.0 w704] -> w181
            tunnel: w180 -> [w209 w246 w306 w407 w488 _ w704]
            tunnel: [w210 w243 w305 w408 w483 w549 w705] -> w179
            tunnel: w178 -> [w210 w244 w305 w408 w481 w549 w705]
            tunnel: [w194 w241 Mode."Plot" ("Enum") Mode."Save" ("Enum") w489 Mode."Return" ("Enum") w701] -> w177
            tunnel: w176 -> [w208 w239 w311 w414 w487 w542 w702]
            tunnel: [w208 w238 w310 w414 w487 w541 w702] -> w175
            tunnel: [w190 FALSE FALSE FALSE w476 TRUE TRUE] -> w174
            tunnel: [w193 w235 w303 w410 w486 0.0 w707] -> w173
            tunnel: w172 -> [w193 w234 w303 w410 w486 _ w707]
            tunnel: w171 -> [_ _ _ _ _ w540 _]
            frame "Offset" {
              n76 = local read "Offset array"() -> (w199:dbl[])
              n77 = local read "Gain (V/A)"() -> (w203:dbl)
              n78 = Unbundle(w205) -> ("read buffer"=w192:string)  [unwired: 2 out]
              n79 = Fract/Exp String To Number(string=w192) -> (number=w204:dbl)  [unwired: 3 in, 1 out]
              n80 = Divide(x=w203, y=1000000000000.0) -> (x/y=w201:dbl)
              n81 = Divide(x=w204, y=w201) -> (x/y=w200:dbl)
              n82 = Build Array (concatenate)(w199, w200) -> (w195:dbl[])
              "Offset array" <- w195
              n83 = Array Size(array=w195) -> (size(s)=w198:i32)
              n84 = Greater?(x=w198, y=100) -> (0:w196:bool)
              n85 = call-poly <vilib>:"Mean.vi"("X"=w195) -> ("mean"=w191:dbl)  [unwired: 1 out]
              "Dc offset" <- w191
              n86 = case shown="False" w196 {
                tunnel: [Mode."Offset" ("Enum") Mode."Process" ("Enum")] -> w194
                tunnel: w191 -> [_ w215]
                tunnel: [TRUE FALSE] -> w190
                frame False {
                }
                frame True {
                  n87 = local read "B/V (T/V)"() -> (w216:dbl)
                  n88 = local read "Gain (V/A)"() -> (w217:dbl)
                  n89 = local read "refnum out"() -> (w221:refnum<file>)
                  n90 = local read "I0 (A)"() -> (w219:dbl)
                  n91 = local read "V/I (Ohm)"() -> (w220:dbl)
                  n92 = local read "B0 (T)"() -> (w218:dbl)
                  n93 = call "File_header_diag.vi"("OFFSET"=w215, "B0"=w218, "B/V"=w216, "I0"=w219, "V/I"=w220, "Gain"=w217, "Byte Stream File in"=w221) -> ()  [unwired: 5 in]
                  n94 = local write "Offset?"(TRUE ("Offset?")) -> ()
                }
              }
            }
            frame "Process", Default {
              # "Converted to pA"
              # "Magnetic Field"
              # "IV converter"
              # "Elapsed Time"
              n95 = local read "Start time"() -> (w258:timestamp)
              n96 = Unbundle(w260) -> ("seconds since 1Jan1904"=w259:timestamp, "read buffer"=w253:string, "read buffer"=w240:string)
              n97 = local read "B/V (T/V)"() -> (w230:dbl)
              n98 = Fract/Exp String To Number(string=w240) -> (number=w250:dbl)  [unwired: 3 in, 1 out]
              n99 = Subtract(x=w259, y=w258) -> (x-y=w235:dbl)
              n100 = Fract/Exp String To Number(string=w253) -> (number=w254:dbl)  [unwired: 3 in, 1 out]
              n101 = Divide(x="Gain (V/A)", y=1000000000000.0) -> (x/y=w233:dbl)
              n102 = Divide(x=w254, y=w233) -> (x/y=w228:dbl)
              n103 = Subtract(x=w235, y=w234) -> (x-y=→"Time Lag":dbl)
              n104 = Build Array (concatenate)(w248, w235) -> (w257:dbl[])
              "Elapsed Time (s)" <- w257
              n105 = local read "Dc offset"() -> (w226:dbl)
              n106 = Subtract(x=w228, y=w226) -> (x-y=w227:dbl)
              "Actual Current (pA)" <- w227
              n107 = Build Array (concatenate)(w255, w227) -> (w256:dbl[])
              "Measured Current (pA)" <- w256
              n108 = local read "B0 (T)"() -> (w229:dbl)
              n109 = xnode "B(U) conversion"("V"=w250, "BpV"=w230, "B0"=w229) -> ("Result"=w249:dbl)  [unwired: 1 in, 1 out]
              "Actual B Field (T)" <- w249
              n110 = Build Array (concatenate)(w251, w249) -> (w252:dbl[])
              "Magnetic Field (T)" <- w252
              n111 = Quotient & Remainder(x=w235, y="Temp Refresh (s)") -> (floor(x/y)=w247:dbl)  [unwired: 1 out]
              n112 = Greater?(x=w247, y=w246) -> (0:w245:bool)
              "Read?" <- w245
              n113 = case shown="True" w245 {
                tunnel: [w266 w281] -> w242
                tunnel: w239 -> [w267 w280]
                tunnel: [w267 w272] -> w238
                tunnel: T5 {"Com Port"=1, "ISOBUS Address"=0, "GPIB Address"=25, "Communication"=enum."GPIB"} ("Address") -> [_ w279]
                tunnel: [w265 w268] -> w224
                frame False {
                  n114 = local read "Setpoint Temperature (K)"() -> (w265:dbl)
                  n115 = local read "Actual Temperature (K)"() -> (w266:dbl)
                }
                frame True {
                  w270 = u32 1000 ("byte count")
                  # "Temperature/Magnet read"
                  n116 = local read "Magnet ON?"() -> (w277:bool)
                  n117 = local read "Lake Shore"() -> (w278:refnum<visa-resource-name>)
                  n118 = case shown="True" w277 {
                    tunnel: w279 -> [_ w285]
                    frame False {
                    }
                    frame True {
                      n119 = call "GPIB - BusCommand.vi"("Command"="R7" ("format string"), "Address"=w285) -> ("Reply"=w286:string)  [unwired: 1 out]
                      n120 = Scan From String(format string="R%f" ("remaining string"), input string=w286) -> (output 1=w284:dbl)  [unwired: 3 in, 3 out]
                      n121 = local write "Actual Field (T)"(w284) -> ()
                    }
                  }
                  n122 = VISA Write(VISA resource name=w278, write buffer="KRDG?a", error in (no error)=w280) -> (VISA resource name out=w271:refnum<visa-resource-name>, error out=w276:errorcluster)  [unwired: 1 out]
                  n123 = VISA Write(VISA resource name=w271, write buffer="SETP?a", error in (no error)=w276) -> (error out=w274:errorcluster)  [unwired: 2 out]
                  n124 = VISA Read(VISA resource name=w271, byte count=w270, error in (no error)=w274) -> (read buffer=w282:string, error out=w273:errorcluster)  [unwired: 2 out]
                  n125 = Fract/Exp String To Number(string=w282) -> (number=w281:dbl)  [unwired: 3 in, 1 out]
                  n126 = VISA Read(VISA resource name=w271, byte count=w270, error in (no error)=w273) -> (VISA resource name out=w269:refnum<visa-resource-name>, error out=w272:errorcluster)  [unwired: 2 out]
                  n127 = Fract/Exp String To Number(string=w269) -> (number=w268:dbl)  [unwired: 3 in, 1 out]
                }
              }
              "Actual Temperature (K)" <- w242
              "Setpoint Temperature (K)" <- w224
              n128 = Build Array (concatenate)(w244, w242) -> (w243:dbl[])
              "Temperature array" <- w243
              n129 = case shown="True" "Sweep" {
                tunnel: [Mode."Plot" ("Enum") Mode."Sweep" ("Enum")] -> w241
                frame False {
                }
                frame True {
                }
              }
            }
            frame "Sweep" {
              n130 = local read "Temp/Magnetic Field"() -> (w301:bool)
              n131 = case shown="True" w301 {
                tunnel: w311 -> [w313 w365]
                tunnel: [w312 w364] -> w310
                frame False {
                  n132 = local read "Actual Field (T)"() -> (w316:dbl)
                  n133 = local read "Min Field (T)"() -> (w315:dbl)
                  n134 = local read "Max Field (T)"() -> (w314:dbl)
                  n135 = local read "Read?"() -> (w319:bool)
                  n136 = Equal?(x=w316, y=w315) -> (x = y?=w317:bool)
                  n137 = And(x=w317, y=w319) -> (x .and. y?=w318:bool)
                  n138 = case shown="True" w318 {
                    tunnel: [w322 w353] -> w312
                    tunnel: w314 -> [w320 w352]
                    tunnel: w315 -> [_ w351]
                    tunnel: w316 -> [_ w349]
                    tunnel: w313 -> [w323 w348]
                    frame True {
                      # "Ramp Up"
                      n139 = case shown="True" "First?" {
                        tunnel: [TRUE ("Save") FALSE ("Save")] -> w326
                        tunnel: [w340 w344] -> w325
                        frame False {
                          n140 = local read "Counter"() -> (w343:i8)
                          n141 = local write "Actual Polarization"(0.0 ("Actual Polarization")) -> ()
                          n142 = Increment(x=w343) -> (x+1=w340:i8)
                          n143 = local write "Counter"(w340) -> ()
                        }
                        frame True {
                          n144 = local read "Counter"() -> (w344:i8)
                          n145 = local write "First?"(FALSE ("First?")) -> ()
                        }
                      }
                      "Reset" <- w326
                      n146 = local write "Read?"(FALSE ("Read?")) -> ()
                      n147 = local read "Record ALL"() -> (w321:bool)
                      n148 = case shown="True" w321 {
                        tunnel: w325 -> [_ w333]
                        tunnel: [FALSE w331] -> w324
                        frame False {
                        }
                        frame True {
                          n149 = Greater?(x=w333, y="Max Countl") -> (0:w331:bool)
                        }
                      }
                      n150 = case shown="True" w324 {
                        tunnel: w323 -> [w336 w339]
                        tunnel: [w335 w339] -> w322
                        tunnel: w320 -> [w334 _]
                        frame False {
                          n151 = call "Set_B.vi"("error in (no error)"=w336, "address string"="25", "Set Field (T)"=w334) -> ("error out"=w335:errorcluster)  [unwired: 8 in]
                        }
                        frame True {
                          "New" <- TRUE
                        }
                      }
                      "Up/Down" <- FALSE ("Up/Down")
                    }
                    frame False {
                      n152 = Equal?(x=w352, y=w349) -> (x = y?=w350:bool)
                      n153 = case shown="True" w350 {
                        tunnel: [w354 w357] -> w353
                        tunnel: w351 -> [_ w355]
                        tunnel: w348 -> [w354 w358]
                        frame False {
                        }
                        frame True {
                          # "Resetting at the end of every cycle"
                          # "Ramp Dn"
                          n154 = local write "Up/Down"(TRUE ("Up/Down")) -> ()
                          n155 = call "Set_B.vi"("error in (no error)"=w358, "address string"="25", "Set Field (T)"=w355) -> ("error out"=w357:errorcluster)  [unwired: 8 in]
                          n156 = local write "Reset"(TRUE ("Reset")) -> ()
                        }
                      }
                      n157 = local write "Read?"(FALSE ("Read?")) -> ()
                    }
                  }
                }
                frame True {
                  n158 = local read "Setpoint Temperature (K)"() -> (w363:dbl)
                  n159 = local read "Min Temperature (K)"() -> (w362:dbl)
                  n160 = local read "Read?"() -> (w368:bool)
                  n161 = local read "Max temperature (K)"() -> (w361:dbl)
                  n162 = Equal?(x=w363, y=w362) -> (x = y?=w366:bool)
                  n163 = And(x=w366, y=w368) -> (x .and. y?=w367:bool)
                  n164 = case shown="False" w367 {
                    tunnel: [w370 w387] -> w364
                    tunnel: w361 -> [w369 w386]
                    tunnel: w362 -> [_ w385]
                    tunnel: w363 -> [_ w383]
                    tunnel: w365 -> [w371 w382]
                    frame True {
                      # "Ramp Up"
                      n165 = local read "First?"() -> (w377:bool)
                      n166 = case shown="False" w377 {
                        frame False {
                          n167 = local read "Counter"() -> (w380:i8)
                          n168 = Increment(x=w380) -> (x+1=w379:i8)
                          n169 = local write "Counter"(w379) -> ()
                        }
                        frame True {
                        }
                      }
                      n170 = local write "Read?"(FALSE ("Read?")) -> ()
                      n171 = Number To Fractional String(number=w369, precision (6)=i16 3) -> (F-format string=w374:string)  [unwired: 2 in]
                      n172 = local read "Lake Shore"() -> (w372:refnum<visa-resource-name>)
                      n173 = Concatenate Strings("SETP 1," ("write buffer"), w374) -> (w376:string)
                      n174 = VISA Write(VISA resource name=w372, write buffer=w376, error in (no error)=w371) -> (error out=w370:errorcluster)  [unwired: 2 out]
                    }
                    frame False {
                      n175 = Equal?(x=w386, y=w383) -> (x = y?=w384:bool)
                      n176 = case shown="True" w384 {
                        tunnel: [w388 w391] -> w387
                        tunnel: w385 -> [_ w390]
                        tunnel: w382 -> [w388 w392]
                        frame False {
                        }
                        frame True {
                          # "Ramp Dn"
                          n177 = local write "Up/Down"(TRUE ("Up/Down")) -> ()
                          n178 = Number To Fractional String(number=w390, precision (6)=i16 3) -> (F-format string=w394:string)  [unwired: 2 in]
                          n179 = local read "Lake Shore"() -> (w389:refnum<visa-resource-name>)
                          n180 = Concatenate Strings("SETP 1," ("write buffer"), w394) -> (w396:string)
                          n181 = VISA Write(VISA resource name=w389, write buffer=w396, error in (no error)=w392) -> (error out=w391:errorcluster)  [unwired: 2 out]
                        }
                      }
                      n182 = local write "Read?"(FALSE ("Read?")) -> ()
                    }
                  }
                }
              }
            }
            frame "Plot" {
              # "dI"
              n183 = local read "P(uC/mm^2)"() -> (w399:dbl[])
              n184 = local read "Actual Polarization"() -> (w398:dbl)
              n185 = local read "Actual Current (pA)"() -> (w400:dbl)
              n186 = local read "Time Lag"() -> (w412:dbl)
              n187 = Multiply(x=w400, y=w412) -> (x*y=w404:dbl)
              n188 = Divide(x=w404, y="Sample area (mm^2)") -> (x/y=w403:dbl)
              n189 = Add(x=w403, y=w398) -> (x+y=w402:dbl)
              "Actual Polarization" <- w402
              n190 = local read "Temp/Magnetic Field"() -> (w413:bool)
              n191 = Build Array (concatenate)(w399, w402) -> (→"P(uC/mm^2)":dbl[])
              n192 = case shown="True" w413 {
                tunnel: w410 -> [_ w473]
                tunnel: w407 -> [_ w455]
                tunnel: w402 -> [w420 w456]
                frame False {
                  # "Magnetic Field plotting"
                  n193 = local read "Up/Down"() -> (w425:bool)
                  n194 = local read "Actual B Field (T)"() -> (w422:dbl)
                  n195 = case shown="False" w425 {
                    frame True {
                      # "Down"
                      n196 = local read "I(B) 3"() -> (w435:cluster{dbl[], dbl[]}[])
                      n197 = local read "I(B) 3"() -> (w439:cluster{dbl[], dbl[]}[])
                      n198 = Index Array(array=w435, index=1) -> (element=w433:cluster{dbl[], dbl[]})
                      n199 = Unbundle(w433) -> (w432:dbl[], w431:dbl[])
                      n200 = Index Array(array=w439, index=i8 0 ("t")) -> (element=w436:cluster{dbl[], dbl[]})
                      n201 = local read "Actual Current (pA)"() -> (w428:dbl)
                      n202 = local read "Actual B Field (T)"() -> (w427:dbl)
                      n203 = Build Array (concatenate)(w432, w427) -> (w430:dbl[])
                      n204 = Build Array (concatenate)(w431, w428) -> (w429:dbl[])
                      n205 = Bundle(w430, w429) -> (w426:cluster{dbl[], dbl[]})  [unwired: 1 in]
                      n206 = Build Array(w436, w426) -> (w437:cluster{dbl[], dbl[]}[])
                      n207 = local write "I(B) 3"(w437) -> ()
                    }
                    frame False {
                      # "Up"
                      n208 = local read "I(B) 3"() -> (w451:cluster{dbl[], dbl[]}[])
                      n209 = local read "I(B) 3"() -> (w453:cluster{dbl[], dbl[]}[])
                      n210 = Index Array(array=w451, index=0) -> (element=w449:cluster{dbl[], dbl[]})
                      n211 = Unbundle(w449) -> (w448:dbl[], w447:dbl[])
                      n212 = Index Array(array=w453, index=i8 1 ("t")) -> (element=w441:cluster{dbl[], dbl[]})
                      n213 = local read "Actual B Field (T)"() -> (w443:dbl)
                      n214 = local read "Actual Current (pA)"() -> (w442:dbl)
                      n215 = Build Array (concatenate)(w448, w443) -> (w446:dbl[])
                      n216 = Build Array (concatenate)(w447, w442) -> (w445:dbl[])
                      n217 = Bundle(w446, w445) -> (w444:cluster{dbl[], dbl[]})  [unwired: 1 in]
                      n218 = Build Array(w444, w441) -> (w440:cluster{dbl[], dbl[]}[])
                      n219 = local write "I(B) 3"(w440) -> ()
                    }
                  }
                  n220 = local read "P(B)"() -> (w424:cluster{"yi":dbl[], dbl[]})
                  n221 = Unbundle(w424) -> ("yi"=w423:dbl[], w421:dbl[])
                  n222 = Build Array (concatenate)(w423, w422) -> (w419:dbl[])
                  n223 = Build Array (concatenate)(w421, w420) -> (w418:dbl[])
                  n224 = Bundle(w419, w418) -> (→"P(B)":cluster{dbl[], dbl[]})  [unwired: 1 in]
                }
                frame True {
                  # "Temperature plotting"
                  n225 = Quotient & Remainder(x=w473, y="Save Period") -> (x-y*floor(x/y)=w454:dbl)  [unwired: 1 out]
                  n226 = Greater?(x=w455, y=w454) -> (0:w471:bool)
                  n227 = local read "Actual Temperature (K)"() -> (w458:dbl)
                  n228 = local read "Actual Current (pA)"() -> (w464:dbl)
                  n229 = local read "P(T)"() -> (w460:cluster{"yi":dbl[], dbl[]})
                  n230 = local read "I(T)"() -> (w470:cluster{dbl[], dbl[]})
                  n231 = case shown="True" w471 {
                    frame False {
                    }
                    frame True {
                      n232 = local write "Reset"(TRUE) -> ()
                    }
                  }
                  n233 = Unbundle(w460) -> ("yi"=w461:dbl[], w457:dbl[])
                  n234 = Unbundle(w470) -> (w468:dbl[], w467:dbl[])
                  n235 = Build Array (concatenate)(w461, w458) -> (w462:dbl[])
                  n236 = Build Array (concatenate)(w457, w456) -> (w463:dbl[])
                  n237 = Build Array (concatenate)(w468, w458) -> (w466:dbl[])
                  n238 = Build Array (concatenate)(w467, w464) -> (w465:dbl[])
                  n239 = Bundle(w466, w465) -> (→"I(T)":cluster{dbl[], dbl[]})  [unwired: 1 in]
                  n240 = Bundle(w462, w463) -> (→"P(T)":cluster{dbl[], dbl[]})  [unwired: 1 in]
                }
              }
            }
            frame "Save" {
              n241 = local read "Reset"() -> (w475:bool)
              n242 = case shown="True" w475 {
                tunnel: w480 -> [w497 w499]
                tunnel: [w497 w502] -> w485
                tunnel: w479 -> [w496 w500]
                tunnel: [w496 w502] -> w484
                tunnel: w481 -> [w495 w501]
                tunnel: [w495 w502] -> w483
                tunnel: [w494 w502] -> w482
                tunnel: w478 -> [w494 w498]
                frame False {
                }
                frame True {
                  n243 = stacked-sequence {
                    tunnel: [_ _ w539] -> w502
                    tunnel: w501 -> [_ w528 _]
                    tunnel: w500 -> [w513 w526 _]
                    tunnel: w499 -> [w514 w527 _]
                    tunnel: w498 -> [_ w524 _]
                    frame #0 {
                      n244 = local read "B array"() -> (w504:dbl[])
                      n245 = local read "Counter"() -> (w512:i8)
                      n246 = local read "Averaged I(B)"() -> (w516:dbl[][])
                      n247 = local read "Up/Down"() -> (w515:bool)
                      n248 = call "Average_IB_curves.vi"("B array"=w504, "Up/Down"=w515, "Counter"=w512, "B in"=w514, "Averaged I(B) In"=w516, "I in"=w513) -> ("Averaged I(B) out"=w507:dbl[][])  [unwired: 5 in]
                      "Averaged I(B)" <- w507
                      n249 = Index Array(array=w507, index (row)=0 ("disabled index (col)")) -> (element=w505:dbl[])  [unwired: 1 in]
                      n250 = Index Array(array=w507, index (row)=1 ("disabled index (col)")) -> (element=w503:dbl[])  [unwired: 1 in]
                      n251 = Bundle("B array"=w504, "Averaged I(B) out"=w505) -> (w511:T7)  [unwired: 1 in]
                      n252 = Bundle("B array"=w504, "Averaged I(B) out"=w503) -> (w510:T7)  [unwired: 1 in]
                      n253 = Build Array(w511, w510) -> (→"I(B) /Averaged/ 2":T8)
                    }
                    frame #1 {
                      # "Save and Reset"
                      n254 = local read "Temp/Magnetic Field"() -> (w517:bool)
                      n255 = local read "Measurement File"() -> (w519:path)
                      n256 = local read "P(uC/mm^2)"() -> (w525:dbl[])
                      n257 = Build Array(w528, w527, w526, w524, w525) -> (w518:dbl[][])
                      n258 = case shown="False" w517 {
                        tunnel: w519 -> [_ _]
                        tunnel: w518 -> [w533 _]
                        frame False {
                          n259 = local read "Up/Down"() -> (w531:bool)
                          n260 = case shown="False" w531 {
                            tunnel: [w536 w537] -> w530
                            frame False {
                              n261 = local read "Measurement File_dn"() -> (w536:path)
                            }
                            frame True {
                              n262 = local read "Measurement File_up"() -> (w537:path)
                            }
                          }
                          n263 = call-poly <vilib>:"Write Delimited Spreadsheet.vi"("file path (dialog if empty)"=w530, "format (%.3f)"="%.5g", "2D data"=w533, "append to file? (F)"=TRUE ("transpose? (F)"), "transpose? (F)"=FALSE ("append to file? (F)")) -> ()  [unwired: 9 in, 2 out]
                        }
                        frame True {
                        }
                      }
                      n264 = case shown="False" "Reset IB?" {
                        frame False {
                        }
                        frame True {
                          n265 = local read "Up/Down"() -> (w538:bool)
                          n266 = case shown="False" w538 {
                            frame False {
                              n267 = invoke on="I(B) 3" class="XYGraph (strict)" method="Reinit To Default"() -> ()  [unwired: 3 in, 3 out]
                            }
                            frame True {
                            }
                          }
                        }
                      }
                      n268 = call-poly <vilib>:"Write Delimited Spreadsheet.vi"("file path (dialog if empty)"=w519, "format (%.3f)"="%.5g", "2D data"=w518, "append to file? (F)"=TRUE, "transpose? (F)"=TRUE) -> ()  [unwired: 9 in, 2 out]
                      n269 = local write "Reset"(FALSE ("Save")) -> ()
                    }
                    frame #2 {
                      w539 = dbl[] []
                      n270 = local write "P(uC/mm^2)"(w539) -> ()
                    }
                  }
                }
              }
              n271 = local read "New"() -> (w477:bool)
              n272 = case shown="True" w477 {
                tunnel: [Mode."Return" ("Enum") Mode."New" ("Enum")] -> w489
                tunnel: [TRUE FALSE] -> w476
                frame False {
                }
                frame True {
                }
              }
            }
            frame "New" {
              n273 = stacked-sequence {
                seq-local: [_ _ _ _ w633 _ _] -> [_ _ _ _ _ w642 _]
                seq-local: [_ _ w587 _ _ _ _] -> [_ _ _ _ w632 _ _]
                tunnel: T5 {"Com Port"=1, "ISOBUS Address"=0, "GPIB Address"=25, "Communication"=enum."GPIB"} ("Address") -> [_ _ w586 w627 _ _ _]
                tunnel: w542 -> [_ _ w588 _ _ w643 _]
                tunnel: [_ _ _ _ _ w645 _] -> w541
                tunnel: w540 -> [_ w567 _ _ _ _ _]
                frame #0 {
                  # "Save averages"
                  n274 = local read "Measurement File_average"() -> (w555:path)
                  n275 = local read "I(B) /Averaged/ 2"() -> (w556:cluster{"B array":dbl[], dbl[]}[])
                  n276 = Index Array(array=w556, index=0) -> (element=w559:cluster{"B array":dbl[], dbl[]})
                  n277 = Index Array(array=w556, index=1) -> (element=w560:cluster{"B array":dbl[], dbl[]})
                  n278 = Unbundle(w559) -> ("B array"=w561:dbl[], w562:dbl[])
                  n279 = Unbundle(w560) -> ("B array"=w563:dbl[], w564:dbl[])
                  n280 = Build Array(w561, w562, w563, w564) -> (w565:dbl[][])
                  n281 = call-poly <vilib>:"Write Delimited Spreadsheet.vi"("file path (dialog if empty)"=w555, "format (%.3f)"="%.5g", "2D data"=w565, "append to file? (F)"=TRUE ("transpose? (F)"), "transpose? (F)"=TRUE ("append to file? (F)")) -> ()  [unwired: 9 in, 2 out]
                }
                frame #1 {
                  w573 = dbl[] []
                  w582 = dbl[] []
                  # "Reset Flags"
                  n282 = Get Date/Time In Seconds() -> (seconds since 1Jan1904=w583:timestamp)
                  n283 = local write "Up/Down"(TRUE ("Up/Down")) -> ()
                  n284 = local write "First?"(TRUE ("First?")) -> ()
                  n285 = local write "Offset?"(FALSE ("Offset?")) -> ()
                  n286 = local write "New"(FALSE ("New")) -> ()
                  n287 = local write "P(uC/mm^2)"(w582) -> ()
                  n288 = local write "Start time"(w583) -> ()
                  n289 = local write "Offset array"(w582) -> ()
                  n290 = local write "Actual Polarization"(0.0 ("Actual Polarization")) -> ()
                  n291 = local write "Up/Down"(TRUE ("Up/Down")) -> ()
                  n292 = local write "Reset"(FALSE ("Reset")) -> ()
                  n293 = local read "B array"() -> (w576:dbl[])
                  n294 = local write "Counter"(i8 0 ("Counter")) -> ()
                  n295 = invoke on="P(B)" class="XYGraph (strict)" method="Reinit To Default"() -> ()  [unwired: 3 in, 3 out]
                  n296 = invoke on="I(B) 3" class="XYGraph (strict)" method="Reinit To Default"() -> ()  [unwired: 3 in, 3 out]
                  n297 = Multiply(x=w576, y=0.0) -> (x*y=w577:dbl[])
                  n298 = Build Array(w573, w573) -> (w581:dbl[][])
                  n299 = Bundle("B array"=w576, w577) -> (w578:cluster{"B array":dbl[], dbl[]})  [unwired: 1 in]
                  n300 = local write "Averaged I(B)"(w581) -> ()
                  n301 = Build Array(w578, w578) -> (w579:cluster{"B array":dbl[], dbl[]}[])
                  n302 = local write "I(B) /Averaged/ 2"(w579) -> ()
                  n303 = local write "Measuring"(FALSE ("Measuring")) -> ()
                  n304 = Flush Queue(queue=w567) -> (remaining elements=→"remaining elements":T1)  [unwired: 1 in, 2 out]
                }
                frame #2 {
                  # "Step"
                  n305 = local read "Sweep Rate Array"() -> (w592:dbl[])
                  n306 = local read "j"() -> (w593:i32)
                  n307 = Increment(x=w593) -> (x+1=w589:i32)
                  n308 = Array Size(array=w592) -> (size(s)=w591:i32)
                  n309 = Less?(x=w589, y=w591) -> (x < y?=w590:bool)
                  "Step Rate" <- w590
                  n310 = case shown="True" w590 {
                    tunnel: w589 -> [_ w620]
                    tunnel: w588 -> [w596 w619]
                    tunnel: [w595 w619] -> w587
                    tunnel: w586 -> [w594 _]
                    frame False {
                      # "Step Temp?"
                      n311 = local read "Temperature Array"() -> (w600:dbl[])
                      n312 = local read "i"() -> (w601:i32)
                      n313 = Increment(x=w601) -> (x+1=w598:i32)
                      n314 = local write "j"(0 ("f")) -> ()
                      n315 = Array Size(array=w600) -> (size(s)=w599:i32)
                      n316 = Less?(x=w598, y=w599) -> (x < y?=w597:bool)
                      "Step Temp" <- w597
                      n317 = case shown="False" w597 {
                        tunnel: w598 -> [_ w618]
                        tunnel: w596 -> [w606 w617]
                        tunnel: [w605 w617] -> w595
                        tunnel: w594 -> [w604 _]
                        frame False {
                          # "Heater OFF"
                          # "Finished"
                          n318 = local write "i"(0 ("i")) -> ()
                          n319 = stacked-sequence {
                            tunnel: w606 -> [w610 _ _]
                            tunnel: [w609 _ _] -> w605
                            tunnel: w604 -> [_ w614 w615]
                            frame #0 {
                              n320 = local read "Lake Shore"() -> (w611:refnum<visa-resource-name>)
                              n321 = VISA Write(VISA resource name=w611, write buffer="RANGE,1,0", error in (no error)=w610) -> (error out=w609:errorcluster)  [unwired: 2 out]
                            }
                            frame #1 {
                              n322 = call "ips_switchHeaterOff.vi"("Instrument address"=w614, "Rate"=2.0) -> ()  [unwired: 1 out]
                            }
                            frame #2 {
                              n323 = call "GPIB - BusCommand.vi"("Command"="H0", "Address"=w615) -> ()  [unwired: 2 out]
                            }
                          }
                          n324 = local write "Record ALL"(FALSE ("Record ALL")) -> ()
                          "Finished" <- TRUE
                        }
                        frame True {
                          n325 = local write "i"(w618) -> ()
                        }
                      }
                    }
                    frame True {
                      n326 = local write "j"(w620) -> ()
                    }
                  }
                }
                frame #3 {
                  # "Set rates"
                  n327 = local read "Sweep Rate Array"() -> (w626:dbl[])
                  n328 = local read "j"() -> (w625:i32)
                  n329 = local read "j"() -> (w623:i32)
                  n330 = Index Array(array=w626, index=w625) -> (element=w624:dbl)
                  n331 = Number To Fractional String(number=w624, precision (6)=i16 3) -> (F-format string=w630:string)  [unwired: 2 in]
                  n332 = Index Array(array="Max count array", index=w623) -> (element=w621:i32)
                  n333 = local write "Max Countl"(w621) -> ()
                  n334 = Concatenate Strings("T" ("format string"), w630) -> (w631:string)
                  n335 = call "GPIB - BusCommand.vi"("Command"=w631, "Address"=w627) -> ()  [unwired: 2 out]
                  n336 = local write "Sweep Rate (T/min)"(w624) -> ()
                }
                frame #4 {
                  # "Set temperature"
                  n337 = local read "Temperature Array"() -> (w636:dbl[])
                  n338 = local read "i"() -> (w635:i32)
                  n339 = Index Array(array=w636, index=w635) -> (element=w634:dbl)
                  n340 = local read "Lake Shore"() -> (w638:refnum<visa-resource-name>)
                  n341 = Number To Fractional String(number=w634, precision (6)=i16 3) -> (F-format string=w639:string)  [unwired: 2 in]
                  n342 = Concatenate Strings("SETP 1," ("write buffer"), w639) -> (w641:string)
                  n343 = VISA Write(VISA resource name=w638, write buffer=w641, error in (no error)=w632) -> (error out=w633:errorcluster)  [unwired: 2 out]
                }
                frame #5 {
                  n344 = local read "Finished"() -> (w644:bool)
                  n345 = case shown="False" w644 {
                    tunnel: [w658 w695] -> w645
                    tunnel: w643 -> [_ _]
                    tunnel: w642 -> [w655 w695]
                    frame False {
                      w653 = "_" ("string")
                      # "Wait, create Files"
                      n346 = local read "Temperature Array"() -> (w685:dbl[])
                      n347 = local read "Sweep Rate Array"() -> (w681:dbl[])
                      n348 = local read "i"() -> (w684:i32)
                      n349 = local read "j"() -> (w682:i32)
                      n350 = Index Array(array=w685, index=w684) -> (element=w683:dbl)
                      n351 = Index Array(array=w681, index=w682) -> (element=w650:dbl)
                      n352 = Round Toward -Infinity(1:w650) -> (0:w651:dbl)
                      n353 = Number To Fractional String(use system decimal point (T)=TRUE, number=w683, precision (6)=i16 1) -> (F-format string=w686:string)  [unwired: 1 in]
                      n354 = Subtract(x=w650, y=w651) -> (x-y=w652:dbl)
                      n355 = Equal To 0?(x=w652) -> (x = 0?=w649:bool)
                      n356 = Select(t=i16 0 ("precision (6)"), s=w649, f=i16 2 ("precision (6)")) -> (s? t:f=w646:i16)
                      n357 = Number To Fractional String(use system decimal point (T)=TRUE, number=w650, precision (6)=w646) -> (F-format string=w654:string)  [unwired: 1 in]
                      n358 = Concatenate Strings("Directory", "\\" ("string"), "FileName", w653, w686, "K" ("string"), w653, w654, "Tpm" ("string")) -> (w675:string)
                      n359 = Search and Replace String(replace all?=TRUE ("replace all? (F)"), input string=w675, search string=".", replace string="p" ("substring (\"\")"), error in=w655) -> (result string=w670:string, error out=w665:errorcluster)  [unwired: 3 in, 2 out]
                      n360 = local write "Step Rate"(FALSE ("Step Rate")) -> ()
                      n361 = Concatenate Strings(w670, ".txt" ("string")) -> (w669:string)
                      n362 = local read "Step Temp"() -> (w659:bool)
                      n363 = String To Path(string=w669) -> (path=w668:path)
                      n364 = Open/Create/Replace File(file path (use dialog)=w668, error in=w665, operation (0:open)=T4."open or create") -> (refnum out=w657:refnum<file>, error out=w658:errorcluster)  [unwired: 3 in, 1 out]
                      n365 = local write "refnum out"(w657) -> ()
                      n366 = Refnum to Path(1:w657) -> (0:w660:path)
                      n367 = call "Create_sweep_files.vi"("Measurement File"=w660) -> ("Path 3"=w663:path, "Path 2"=w662:path, "Path"=w661:path)  [unwired: 8 in]
                      n368 = local write "Measurement File"(w660) -> ()
                      n369 = case shown="True" w659 {
                        frame False {
                        }
                        frame True {
                          n370 = Get Date/Time In Seconds() -> (seconds since 1Jan1904=w688:timestamp)
                          n371 = local write "Step Temp"(FALSE ("Step Temp")) -> ()
                          n372 = while {
                            tunnel: w688 -> [w693]
                            stop <- w690 stop-if-true
                            n373 = Get Date/Time In Seconds() -> (seconds since 1Jan1904=w694:timestamp)
                            n374 = Subtract(x=w694, y=w693) -> (x-y=w692:dbl)
                            "Wait (s)" <- w692
                            n375 = Greater Or Equal?(x=w692, y="secs to wait") -> (x >= y?=w690:bool)
                          }
                        }
                      }
                      n376 = local write "Measurement File_dn"(w663) -> ()
                      n377 = local write "Measurement File_average"(w661) -> ()
                      n378 = local write "Measurement File_up"(w662) -> ()
                    }
                    frame True {
                    }
                  }
                }
                frame #6 {
                  n379 = local read "Finished"() -> (w696:bool)
                  n380 = case shown="True" w696 {
                    frame False {
                      n381 = local write "Measuring"(TRUE ("Measuring")) -> ()
                    }
                    frame True {
                      n382 = local write "Measure /Pause"(FALSE ("Measure /Pause")) -> ()
                    }
                  }
                }
              }
            }
            frame "Return" {
            }
          }
        }
      }
      frame Error {
        # "Return true for any case which should stop the loop."
      }
    }
  }
  n383 = case shown="True" w26 {
    frame False {
    }
    frame True {
      n384 = invoke on="P(T)" class="XYGraph (strict)" method="Reinit To Default"() -> ()  [unwired: 3 in, 3 out]
      n385 = invoke on="I(T)" class="XYGraph (strict)" method="Reinit To Default"() -> ()  [unwired: 3 in, 3 out]
    }
  }
  n386 = while {
    shift-right: [w727] -> w70
    shift-left: w49 -> [w728]
    shift-right: [w729] -> w77
    shift-left: w78 -> [w730]
    tunnel: w73 -> [w726]
    tunnel: w72 -> [w725]
    tunnel: w12 -> [w724]
    tunnel: [w718] -> _
    tunnel: w58 -> [w717]
    tunnel: w47 -> [w716]
    stop <- "stop" stop-if-true
    n387 = event shown="[11] \"Heater On/Off\": Value Change" {
      selector: _ -> [_ _ _ _ _ _ _ _ _ _ _ _ _ _ _]
      dyn-events: _ -> [_ _ _ _ _ _ _ _ _ _ _ _ _ _ _]
      timeout: 10 -> [_ _ _ _ _ _ _ _ _ _ _ _ _ _ _]
      tunnel: w730 -> [w740 w772 w781 w789 w800 w805 w809 w835 w851 w868 w911 w928 w944 w954 w965]
      tunnel: [w739 w772 w781 w789 w800 w805 w809 w835 w851 w868 w911 w928 w944 w954 w965] -> w729
      tunnel: w728 -> [w738 w771 w780 w790 w799 w807 w811 w836 w850 w867 w912 w930 w948 w958 w967]
      tunnel: [w737 w771 w780 w790 w801 w807 w810 _ w850 w867 w912 w929 w947 w957 w966] -> w727
      tunnel: w726 -> [w736 _ _ _ _ _ _ _ _ _ _ _ _ _ _]
      tunnel: w725 -> [w735 _ _ _ _ _ _ _ _ _ _ _ _ _ _]
      tunnel: w724 -> [w734 _ _ _ _ _ _ _ _ _ _ _ _ _ _]
      tunnel: [w732 w770 w779 w788 w802 w806 w808 w834 w849 w866 w910 w927 w945 w955 _] -> w718
      tunnel: w717 -> [w732 w770 w782 w788 w802 w806 w808 w834 w849 w866 w910 w927 w945 w955 _]
      tunnel: w716 -> [_ _ _ _ _ _ _ _ _ _ _ w931 w946 w959 w964]
      tunnel: [_ _ _ _ _ _ _ w836 _ _ _ _ _ _ _] -> _
      event Timeout {
        n388 = event-data() -> ()  [unwired: 1 in, 3 out]
        n389 = case shown="True" "Measuring" {
          tunnel: w740 -> [w742 w761]
          tunnel: [w742 w760] -> w739
          tunnel: w738 -> [w741 _]
          tunnel: [w741 w759] -> w737
          tunnel: w736 -> [_ w752]
          tunnel: w735 -> [_ w751]
          tunnel: w734 -> [_ w746]
          frame False {
          }
          frame True {
            w749 = ":FETCh? " ("data")
            w753 = u32 1000 ("byte count")
            # "Generate the data here."
            n390 = case shown="No Error" w746 {
              selector: w746 -> [w763 w764]
              tunnel: [w763 w764] -> w745
              tunnel: [w762 _] -> w744
              frame No Error {
                n391 = Get Date/Time In Seconds() -> (seconds since 1Jan1904=w762:timestamp)
              }
              frame Error {
              }
            }
            n392 = VISA Write(VISA resource name=w752, write buffer=w749, error in (no error)=w745) -> (VISA resource name out=w758:refnum<visa-resource-name>, error out=w756:errorcluster)  [unwired: 1 out]
            n393 = VISA Write(VISA resource name=w751, write buffer=w749, error in (no error)=w756) -> (VISA resource name out=w757:refnum<visa-resource-name>, error out=w755:errorcluster)  [unwired: 1 out]
            n394 = VISA Read(VISA resource name=w758, byte count=w753, error in (no error)=w755) -> (read buffer=w747:string, error out=w754:errorcluster)  [unwired: 2 out]
            n395 = VISA Read(VISA resource name=w757, byte count=w753, error in (no error)=w754) -> (read buffer=w748:string, error out=w750:errorcluster)  [unwired: 2 out]
            n396 = Bundle("seconds since 1Jan1904"=w744, "read buffer"=w747, "read buffer"=w748) -> (w743:T6)  [unwired: 1 in]
            n397 = Enqueue Element(queue=w761, element=w743, error in (no error)=w750) -> (queue out=w760:refnum<queue>, error out=w759:errorcluster)  [unwired: 1 in, 1 out]
          }
        }
      }
      event "Max Field (T)": Value Change {
        n398 = event-data() -> ()  [unwired: 1 in, 6 out]
        n399 = Divide(x="Max Field (T)", y="dB (T)") -> (x/y=w767:dbl)
        n400 = for {
          N: w767 -> [_]
          tunnel: "dB (T)" -> [w777]
          tunnel: [w774] -> w766 mode=indexing
          tunnel: "Min Field (T)" -> [w775]
          tunnel: [0.0] -> _ mode=indexing
          i -> [w778]
          n401 = Multiply(x=w778, y=w777) -> (x*y=w776:dbl)
          n402 = Add(x=w776, y=w775) -> (x+y=w774:dbl)
        }
        "B array" <- w766
      }
      event "Sweep Rate (T/min)": Value Change {
        n403 = event-data() -> ("NewVal"=w786:dbl)  [unwired: 1 in, 5 out]
        n404 = Number To Fractional String(number=w786, precision (6)=i16 3) -> (F-format string=w784:string)  [unwired: 2 in]
        n405 = Concatenate Strings("T" ("format string"), w784) -> (w783:string)
        n406 = call "GPIB - BusCommand.vi"("Command"=w783, "Address"=w782) -> ("Address(thru)"=w779:T5)  [unwired: 1 out]
      }
      event "Field To Zero": Value Change {
        n407 = event-data() -> ()  [unwired: 1 in, 6 out]
        n408 = Two Button Dialog(message="Do you want to switch off the field?", 1:"No" ("F button name (\"Cancel\")"), 2:"Yes" ("T button name (\"OK\")")) -> (T button?=w794:bool)
        n409 = case shown="True" w794 {
          tunnel: w788 -> [_ w797]
          frame False {
          }
          frame True {
            n410 = local read "Sweep Rate (T/min)"() -> (w796:dbl)
            n411 = call "ips_switchHeaterOff.vi"("Instrument address"=w797, "Rate"=w796) -> ("B"=w795:dbl)
            n412 = local write "Actual Field (T)"(w795) -> ()
          }
        }
      }
      event "Go to Set": Value Change {
        n413 = event-data() -> ()  [unwired: 1 in, 6 out]
        n414 = call "Set_B.vi"("error in (no error)"=w799, "address string"="25", "Set Field (T)"="Set Field (T)") -> ("error out"=w801:errorcluster)  [unwired: 8 in]
      }
      event "Measure /Pause": Value Change {
        n415 = event-data() -> ("NewVal"=w804:bool)  [unwired: 1 in, 5 out]
        n416 = local write "Measuring"(w804) -> ()
      }
      event "Stop": Value Change {
        n417 = event-data() -> ()  [unwired: 1 in, 6 out]
        n418 = local read "Measuring"() -> (w812:bool)
        n419 = case shown="True" w812 {
          tunnel: w811 -> [w813 w816]
          tunnel: [w813 w815] -> w810
          frame False {
          }
          frame True {
            w814 = FALSE ("Measuring")
            n420 = local read "SaveSweep"() -> (w819:bool)
            n421 = local write "Measuring"(w814) -> ()
            n422 = local read "Set Field (T)"() -> (w817:dbl)
            n423 = local write "Measure /Pause"(w814) -> ()
            n424 = case shown="True" w819 {
              frame False {
              }
              frame True {
                n425 = local read "Measurement File_average"() -> (w830:path)
                n426 = local read "I(B) /Averaged/ 2"() -> (w829:cluster{"B array":dbl[], dbl[]}[])
                n427 = Index Array(array=w829, index=0) -> (element=w826:cluster{"B array":dbl[], dbl[]})
                n428 = Index Array(array=w829, index=1) -> (element=w825:cluster{"B array":dbl[], dbl[]})
                n429 = Unbundle(w826) -> ("B array"=w824:dbl[], w823:dbl[])
                n430 = Unbundle(w825) -> ("B array"=w822:dbl[], w821:dbl[])
                n431 = Build Array(w824, w823, w822, w821) -> (w820:dbl[][])
                n432 = call-poly <vilib>:"Write Delimited Spreadsheet.vi"("file path (dialog if empty)"=w830, "format (%.3f)"="%.5g", "2D data"=w820, "append to file? (F)"=TRUE ("transpose? (F)"), "transpose? (F)"=TRUE ("append to file? (F)")) -> ()  [unwired: 9 in, 2 out]
              }
            }
            n433 = call "Set_B.vi"("error in (no error)"=w816, "address string"="25", "Set Field (T)"=w817) -> ("error out"=w815:errorcluster)  [unwired: 8 in]
          }
        }
      }
      event "Sweep": Value Change {
        n434 = event-data() -> ("NewVal"=w837:bool)  [unwired: 1 in, 5 out]
        n435 = case shown="True" w837 {
          frame False {
          }
          frame True {
            n436 = local read "Measurement File"() -> (w838:path)
            n437 = Two Button Dialog(message="Do you want to create additional files for the sweeping measurements?" ("string"), 1:"No" ("F button name (\"Cancel\")"), 2:"Yes" ("T button name (\"OK\")")) -> (T button?=w840:bool)
            n438 = case shown="True" w840 {
              tunnel: w838 -> [_ w845]
              frame False {
                n439 = local write "SaveSweep"(FALSE ("SaveSweep")) -> ()
              }
              frame True {
                n440 = call "Create_sweep_files.vi"("Measurement File"=w845) -> ("Path 3"=→"Measurement File_dn":path, "Path 2"=→"Measurement File_up":path, "Path"=→"Measurement File_average":path)  [unwired: 8 in]
                "SaveSweep" <- TRUE
              }
            }
          }
        }
      }
      event "Measure Noise": Value Change {
        n441 = event-data() -> ("NewVal"=w852:bool)  [unwired: 1 in, 5 out]
        n442 = case shown="True" w852 {
          frame False {
          }
          frame True {
            n443 = local read "Gain (V/A)"() -> (w857:dbl)
            n444 = call "Noise_measurement.vi"("Gain (V/A)"=w857, "Cycles"="Cycles", "Lower Cut-Off"="Cut-Off Frequency", "minimum value"="minimum value", "Filter On"="Filter On", "maximum value"="maximum value", "physical channels"="physical channels", "rate"="Rate", "samples per channel"="Samples per channel") -> ("Current (pA) Filtered"=→"Current (pA) Filtered":waveform(dbl), "PSD (pA/Hz^1/2) Peaks Removed"=→"PSD (pA/Hz^1/2) Peaks Removed":cluster{"f0":dbl, "df":dbl, "magnitude":dbl[]}, "Current (pA)"=→"Current (pA)":dbl[], "PSD (pA/Hz^1/2)"=→"PSD (pA/Hz^1/2)":cluster{"f0":dbl, "df":dbl, "magnitude":dbl[]})  [unwired: 3 in]
          }
        }
      }
      event "Calibrate": Value Change {
        n445 = event-data() -> ()  [unwired: 1 in, 6 out]
        n446 = case shown="True" "Calibrate" {
          frame False {
          }
          frame True {
            w872 = dbl[] []
            n447 = while {
              shift-right: [w905] -> w870
              shift-left: dbl[][] [] -> [w904]
              shift-right: [w888] -> _
              shift-left: w872 -> [w900]
              shift-right: [w897] -> _
              shift-left: w872 -> [w899]
              shift-right: [w887] -> _
              shift-left: w872 -> [w898]
              shift-right: [w879] -> _
              shift-left: 0.0 ("Set Field out") -> [w878]
              stop <- w901 stop-if-true
              n448 = call "Calibtarion.vi"("Dwell Time (ms)"="Dwell Time (ms)", "V array in (V)"=w900, "I array in (A)"=w898, "Collected array in"=w904, "B array in (T)"=w899, "Set Field (T)"=w878, "dB"="dB") -> ("Best Linear Fit"=w889:dbl[], "appended array"=→"appended array":dbl[][], "slope"=→"B/V (T/V)":dbl, "V array out (V)"=w888:dbl[], "Boolean"=w903:bool, "I array out (A)"=w887:dbl[], "intercept 2"=→"I0 (A)":dbl, "Collected array out"=w905:dbl[][], "intercept"=→"B0 (T)":dbl, "B array Out"=w897:dbl[], "slope 2"=→"V/I (Ohm)":dbl, "Best Linear Fit 2"=w894:dbl[], "Set Field out"=w879:dbl)
              n449 = Bundle("I array out (A)"=w887, "V array out (V)"=w888) -> (w896:T9)  [unwired: 1 in]
              n450 = Bundle("I array out (A)"=w887, "Best Linear Fit"=w889) -> (w890:T10)  [unwired: 1 in]
              n451 = Bundle("V array out (V)"=w888, "B array Out"=w897) -> (w892:T11)  [unwired: 1 in]
              n452 = Bundle("V array out (V)"=w888, "Best Linear Fit 2"=w894) -> (w893:T12)  [unwired: 1 in]
              n453 = Or(x=w903, y="stop 2") -> (x .or. y?=w901:bool)
              n454 = Build Array(w896, w890) -> (→"V_I":T13)
              n455 = Build Array(w892, w893) -> (→"B_V":T14)
            }
            n456 = flat-sequence {
              tunnel: w870 -> [w876]
              frame #0 {
                n457 = Two Button Dialog(message="Do you want to save calibration file?") -> (T button?=w875:bool)  [unwired: 2 in]
                n458 = case shown="True" w875 {
                  tunnel: w876 -> [_ w877]
                  frame False {
                  }
                  frame True {
                    n459 = call-poly <vilib>:"Write Delimited Spreadsheet.vi"("2D data"=w877) -> ()  [unwired: 13 in, 2 out]
                  }
                }
              }
            }
          }
        }
      }
      event "New Measurement File": Value Change {
        n460 = event-data() -> ()  [unwired: 1 in, 6 out]
        n461 = local read "Sweep"() -> (w907:bool)
        n462 = Open/Create/Replace File(prompt="Please select measurement file\n", operation (0:open)=T4."replace or create with confirmation") -> (refnum out=w913:refnum<file>)  [unwired: 4 in, 2 out]
        n463 = local write "refnum out"(w913) -> ()
        n464 = Refnum to Path(1:w913) -> (0:w908:path)
        n465 = case shown="True" w907 {
          tunnel: w908 -> [_ w916]
          frame False {
          }
          frame True {
            n466 = Two Button Dialog(message="Do you want to create additional files for the sweeping measurements?" ("string"), 1:"No" ("F button name (\"Cancel\")"), 2:"Yes" ("T button name (\"OK\")")) -> (T button?=w918:bool)
            n467 = case shown="False" w918 {
              tunnel: w916 -> [_ w926]
              frame False {
                n468 = local write "SaveSweep"(FALSE ("SaveSweep")) -> ()
              }
              frame True {
                n469 = call "Create_sweep_files.vi"("Measurement File"=w926) -> ("Path 3"=w923:path, "Path 2"=w924:path, "Path"=w925:path)  [unwired: 8 in]
                n470 = local write "Measurement File_dn"(w923) -> ()
                n471 = local write "Measurement File_average"(w925) -> ()
                n472 = local write "Measurement File_up"(w924) -> ()
                n473 = local write "SaveSweep"(TRUE) -> ()
              }
            }
          }
        }
        n474 = local write "Measurement File"(w908) -> ()
        n475 = local write "Offset?"(FALSE ("Offset?")) -> ()
        n476 = local write "First?"(TRUE ("First?")) -> ()
      }
      event "Heater On/Off": Value Change {
        n477 = event-data() -> ()  [unwired: 1 in, 6 out]
        n478 = case shown="False" "Heater On/Off" {
          tunnel: w931 -> [w936 w942]
          tunnel: w930 -> [w934 w943]
          tunnel: [w933 w941] -> w929
          frame False {
            n479 = VISA Write(VISA resource name=w936, write buffer="RANGE,1,0", error in (no error)=w934) -> (error out=w933:errorcluster)  [unwired: 2 out]
          }
          frame True {
            n480 = Number To Decimal String(number="Heater Range") -> (decimal integer string=w939:string)  [unwired: 1 in]
            n481 = Concatenate Strings("RANGE,1," ("write buffer"), w939) -> (w937:string)
            n482 = VISA Write(VISA resource name=w942, write buffer=w937, error in (no error)=w943) -> (error out=w941:errorcluster)  [unwired: 2 out]
          }
        }
      }
      event "Set temperature (K)": Value Change {
        n483 = event-data() -> ()  [unwired: 1 in, 6 out]
        n484 = local read "Set temperature (K)"() -> (w949:dbl)
        n485 = Number To Fractional String(number=w949, precision (6)=i16 3) -> (F-format string=w952:string)  [unwired: 2 in]
        n486 = Concatenate Strings("SETP 1," ("write buffer"), w952) -> (w950:string)
        n487 = VISA Write(VISA resource name=w946, write buffer=w950, error in (no error)=w948) -> (error out=w947:errorcluster)  [unwired: 2 out]
      }
      event "Temp Ramping Rate (K/min)": Value Change {
        n488 = event-data() -> ()  [unwired: 1 in, 6 out]
        n489 = local read "Temp Ramping Rate (K/min)"() -> (w956:dbl)
        n490 = Number To Fractional String(number=w956, precision (6)=i16 1) -> (F-format string=w962:string)  [unwired: 2 in]
        n491 = Concatenate Strings("RAMP 1,1," ("string"), w962) -> (w961:string)
        n492 = VISA Write(VISA resource name=w959, write buffer=w961, error in (no error)=w958) -> (error out=w957:errorcluster)  [unwired: 2 out]
      }
      event "Heater Range": Value Change {
        n493 = event-data() -> ()  [unwired: 1 in, 6 out]
        n494 = local read "Heater On/Off"() -> (w968:bool)
        n495 = case shown="True" w968 {
          tunnel: w967 -> [w969 w974]
          tunnel: [w969 w973] -> w966
          tunnel: w964 -> [_ w972]
          frame False {
          }
          frame True {
            n496 = local read "Heater Range"() -> (w970:enum16{"Off", "Low", "Medium", "High"})
            n497 = Number To Decimal String(number=w970) -> (decimal integer string=w976:string)  [unwired: 1 in]
            n498 = Concatenate Strings("RANGE,1," ("write buffer"), w976) -> (w975:string)
            n499 = VISA Write(VISA resource name=w972, write buffer=w975, error in (no error)=w974) -> (error out=w973:errorcluster)  [unwired: 2 out]
          }
        }
      }
    }
    n500 = Reciprocal(x="Sampling rate (Hz)") -> (1/x=w722:dbl)
    n501 = Multiply(x=w722, y=1000.0) -> (x*y=w720:dbl)
    n502 = Wait Until Next ms Multiple(millisecond multiple=w720) -> ()  [unwired: 1 out]
  }
  n503 = local read "Max Field (T)"() -> (w36:dbl)
  n504 = local read "Min Field (T)"() -> (w38:dbl)
  n505 = local read "dB (T)"() -> (w37:dbl)
  n506 = Divide(x=w36, y=w37) -> (x/y=w39:dbl)
  n507 = for {
    N: w39 -> [_]
    tunnel: w37 -> [w981]
    tunnel: [w978] -> w35 mode=indexing
    tunnel: w38 -> [w979]
    tunnel: [0.0] -> _ mode=indexing
    i -> [w982]
    n508 = Multiply(x=w982, y=w981) -> (x*y=w980:dbl)
    n509 = Add(x=w980, y=w979) -> (x+y=w978:dbl)
  }
  n510 = local write "B array"(w35) -> ()
  n511 = local read "Lake Shore"() -> (w50:refnum<visa-resource-name>)
  n512 = local read "IV converter"() -> (w68:refnum<visa-resource-name>)
  n513 = local read "Magnetic Field"() -> (w67:refnum<visa-resource-name>)
  n514 = VISA Close(VISA resource name=w68, error in (no error)=w70) -> (error out=w71:errorcluster)
  n515 = VISA Close(VISA resource name=w67, error in (no error)=w71) -> (error out=w69:errorcluster)
  n516 = Release Queue(queue=w77, error in (no error)=w69) -> (error out=w64:errorcluster)  [unwired: 1 in, 2 out]
  n517 = Merge Errors(w64, w63) -> (w65:errorcluster)
  n518 = VISA Close(VISA resource name=w50, error in (no error)=w65) -> (error out=w62:errorcluster)
  n519 = local read "refnum out"() -> (w60:refnum<file>)
  n520 = Close File(refnum=w60, error in=w62) -> (error out=w61:errorcluster)  [unwired: 1 out]
  n521 = call <vilib>:"Simple Error Handler.vi"("error in (no error)"=w61) -> ()  [unwired: 4 in, 5 out]
  "i" <- w27
  "j" <- w27
